vi "EXPERIMENTAL_OSCILLOSCOPE_READING.vi"() -> ()   [LabVIEW 2019]
uses:
  <instrlib>/niScope/Controls/niScope vertical coupling.ctl
  Controls/OscilloscopeBlockControl2.ctl
  Controls/DataBlockControl.ctl
  <instrlib>/niScope/Acquire/Fetch/niScope Multi Fetch Binary 16.vi
panel:
  in  "New Run?":bool=TRUE
  in  "Reset Value attempt 2":i32
  in  "Plot Data attempt 2":bool
  in  "Oscilloscope Config Cluster":T1 {"vertical coupling" items=["AC", "DC", "Ground"]}
  in  "error in":errorcluster
  in  "Oscilloscope Configuration Input Array":T1[](array[typedef]) {"vertical coupling" items=["AC", "DC", "Ground"]}
  out "Channel Graph 7":dbl[](graph)
  out "Channel Graph 6":dbl[](graph)
  out "Channel Graph 5":dbl[](graph)
  out "Channel Graph 4":dbl[](graph)
  out "Channel Graph 3":dbl[](graph)
  out "Channel Graph 2":dbl[](graph)
  out "Channel Graph 1":dbl[](graph)
  out "Channel Graph 0":dbl[](graph)
  out "Pryor's Graph":dbl[][](graph)
  in  "Plot Data":bool
  in  "Reset Value":i32=251
  in  "element":T3 {"vertical coupling" items=["AC", "DC", "Ground"]}
  in  "Oscilloscope Configuration Input Array":T4(array[cluster]) {"vertical coupling" items=["AC", "DC", "Ground"]}
  out "end record":bool
  out "error out":errorcluster
  in  "stop":bool
  out "Sample Rate IND":dbl
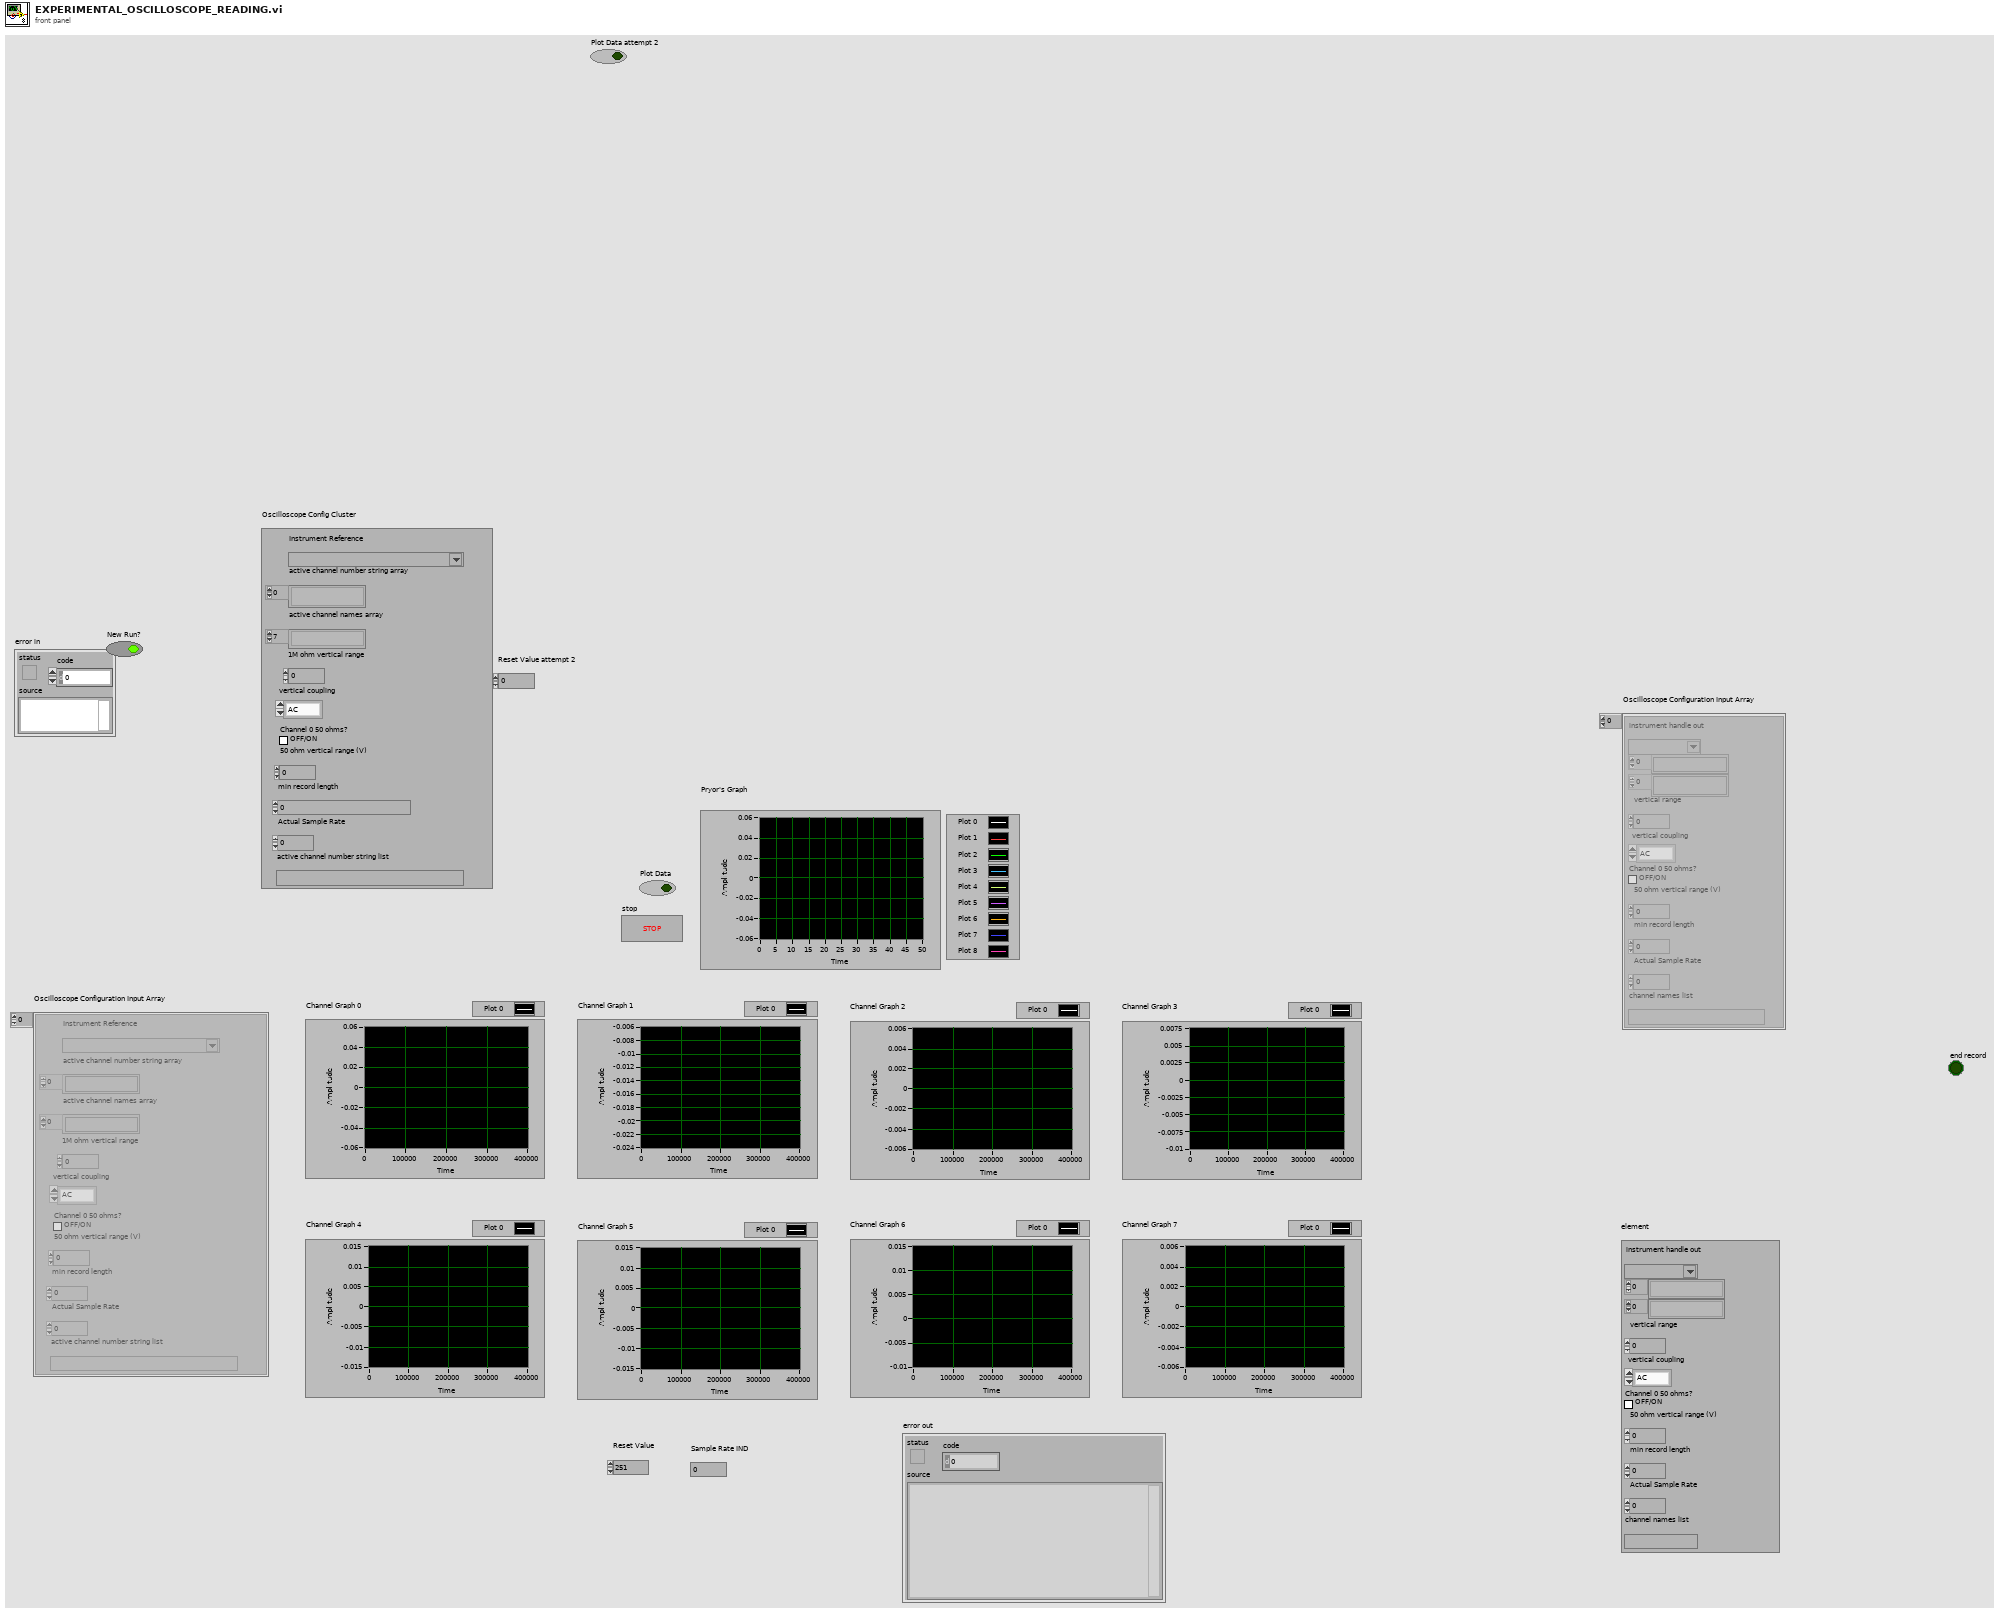
[diagram p1: front panel]
types:
  T1 = typedef "OscilloscopeBlockControl2.ctl" = cluster{"Instrument Reference":refnum<k15>, "active channel number string array":string[], "active channel names array":string[], "1M ohm vertical range":dbl, "vertical coupling":T2, "Channel 0 50 ohms?":bool, "50 ohm vertical range (V)":dbl, "min record length":i32, "Actual Sample Rate":dbl, "active channel number string list":string}
  T2 = typedef "niScope vertical coupling.ctl" = i32
  T3 = cluster{"instrument handle out":refnum<k15>, string[], string[], "vertical range":dbl, "vertical coupling":T2, "Channel 0 50 ohms?":bool, "50 ohm vertical range (V)":dbl, "min record length":i32, "Actual Sample Rate":dbl, "channel names list":string}
  T4 = cluster{"instrument handle out":refnum<k15>, string[], string[], "vertical range":dbl, "vertical coupling":T2, "Channel 0 50 ohms?":bool, "50 ohm vertical range (V)":dbl, "min record length":i32, "Actual Sample Rate":dbl, "channel names list":string}[]
  T5 = cluster{"IVI Refnum out":refnum<k15>, string, "voltage level channel 23":dbl, "Channel Name 23":string, "Current Limit":dbl, "Measure Record dt":dbl, string}[]
  T6 = typedef "DataBlockControl.ctl" = cluster{"Run Folder Parent Directory":path, "DUT":string, "Ion (ex Kr)":string, "Board Number":string, "Effective LET":string, "Test Type":enum16{"Single Event Latchup", "Single Event Transient", "Single Event Upset"}}
  T7 = enum16{"open", "replace", "create", "open or create", "replace or create", "replace or create with confirmation"}
  T8 = cluster{"Array":dbl[], "Array":dbl[], "Array":dbl[], "Array":dbl[], "Array":dbl[], "Array":dbl[], "Array":dbl[], "Array":dbl[]}
  T9 = cluster{"wfm info":cluster{"actualSamples":i32, "absoluteInitialX":dbl, "relativeInitialX":dbl, "xIncrement":dbl, "offset":dbl, "gain":dbl, "reserved1":dbl, "reserved2":dbl}[], "wfm":i16[][]}
  T10 = cluster{"created path":path, refnum<file>[], refnum<file>[]}
  T11 = enum16{"big-endian, network order", "native, host order", "little-endian"}
  T12 = cluster{"actualSamples":i32, "absoluteInitialX":dbl, "relativeInitialX":dbl, "xIncrement":dbl, "offset":dbl, "gain":dbl, "reserved1":dbl, "reserved2":dbl}[]
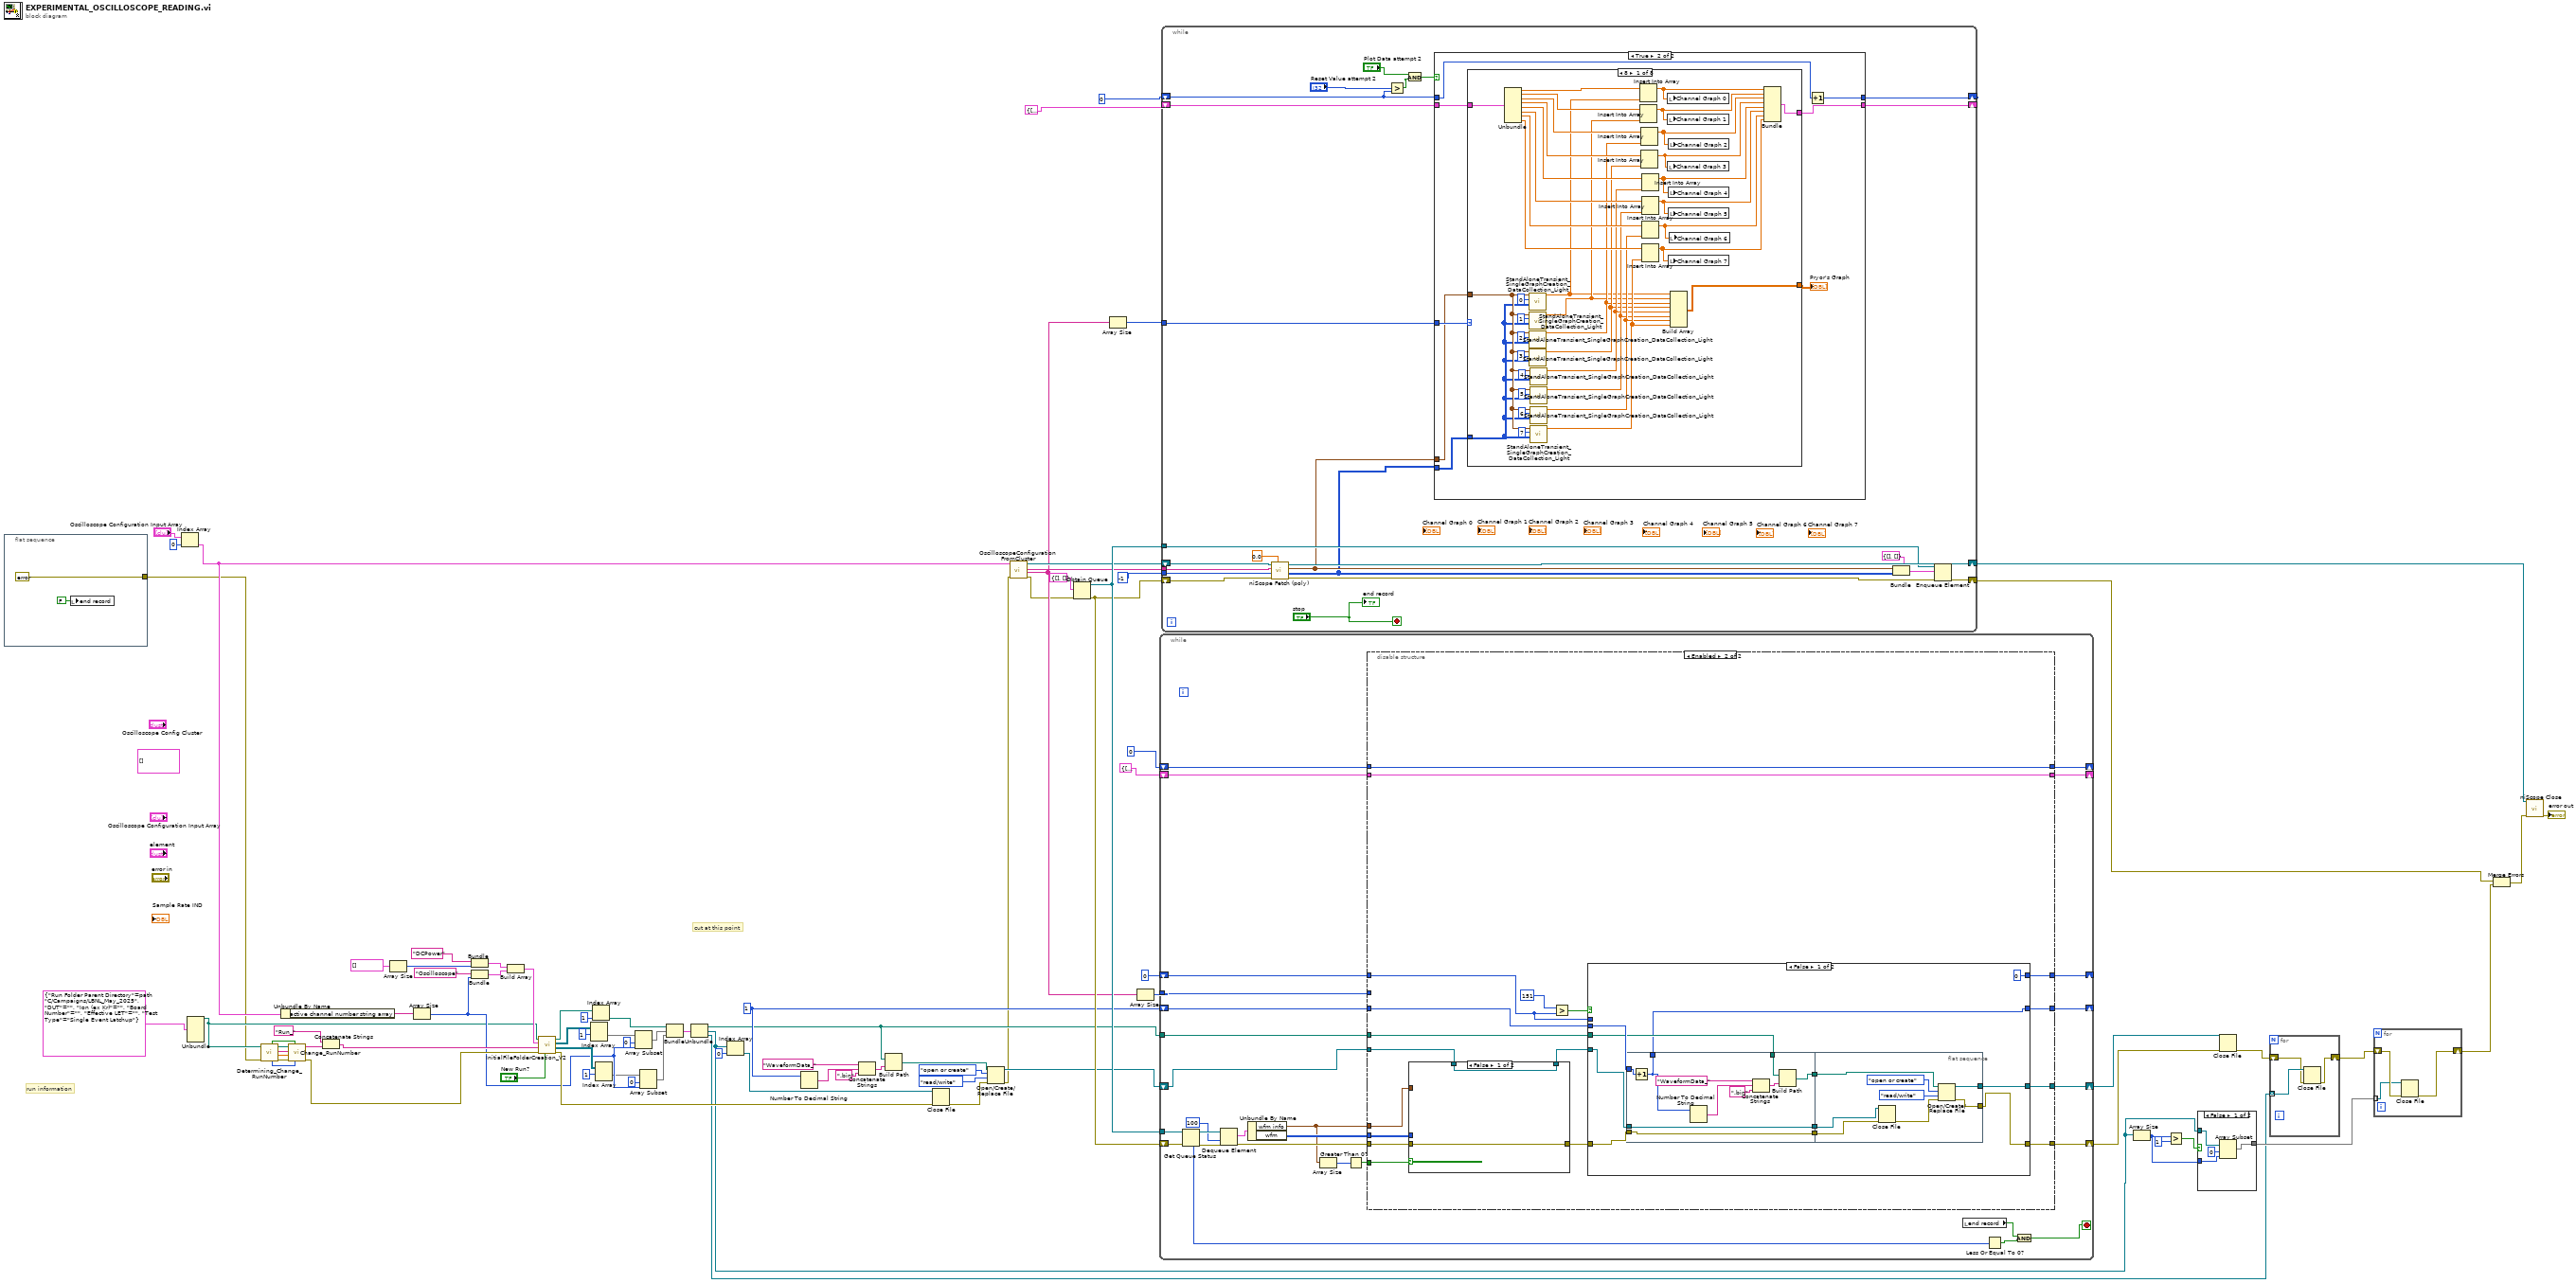
[diagram p0: block diagram]
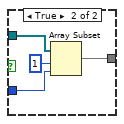
[diagram p2: hidden frame]
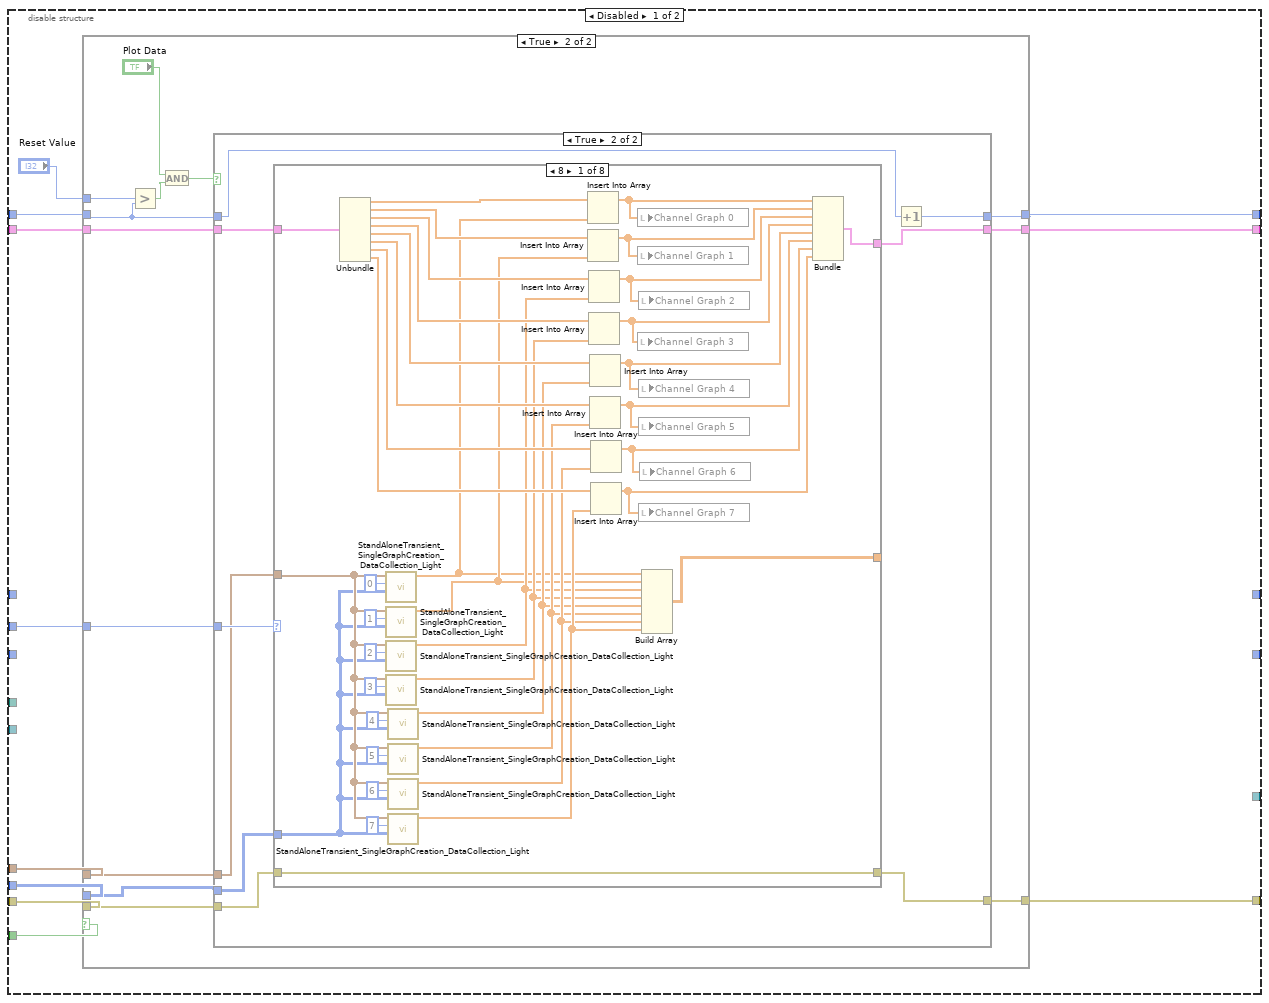
[diagram p3: hidden frame]
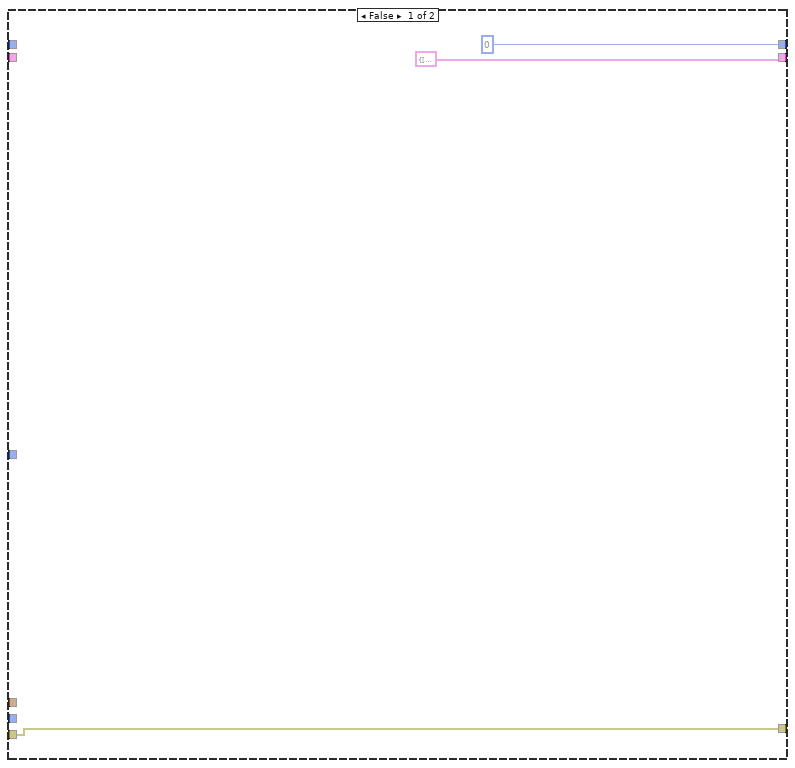
[diagram p5: hidden frame]
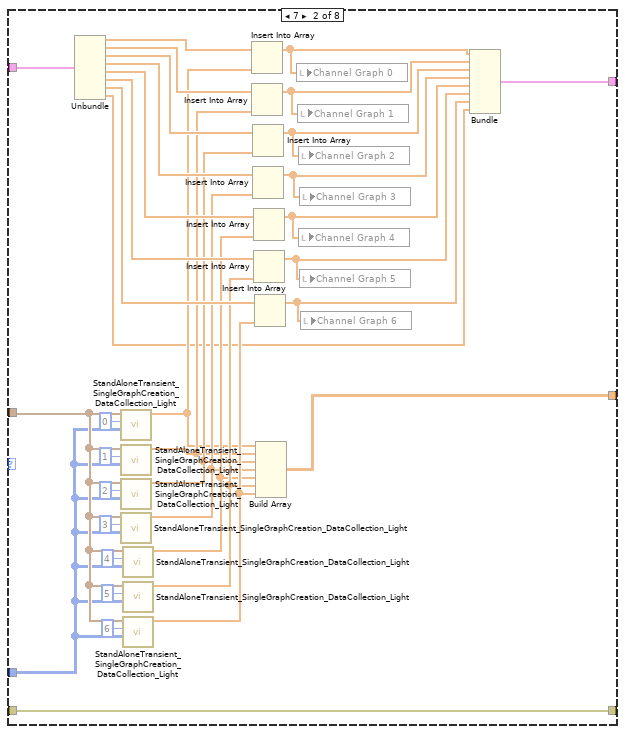
[diagram p6: hidden frame]
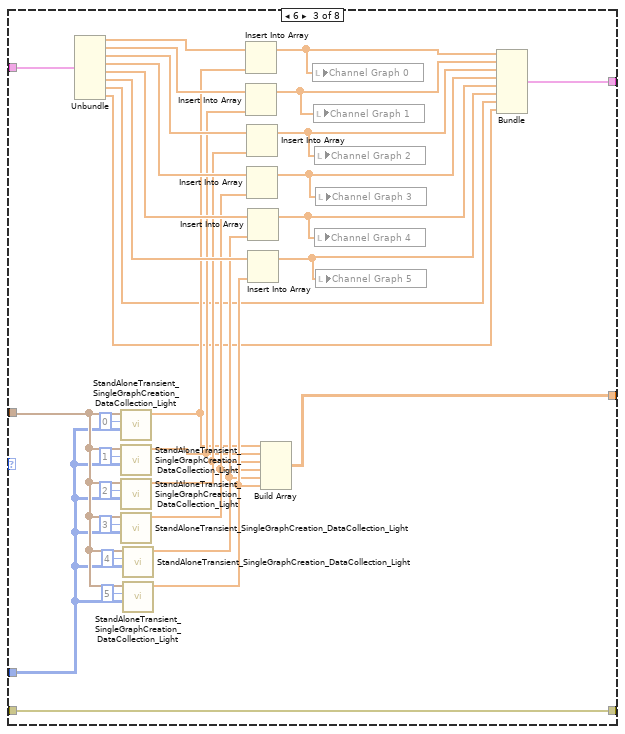
[diagram p7: hidden frame]
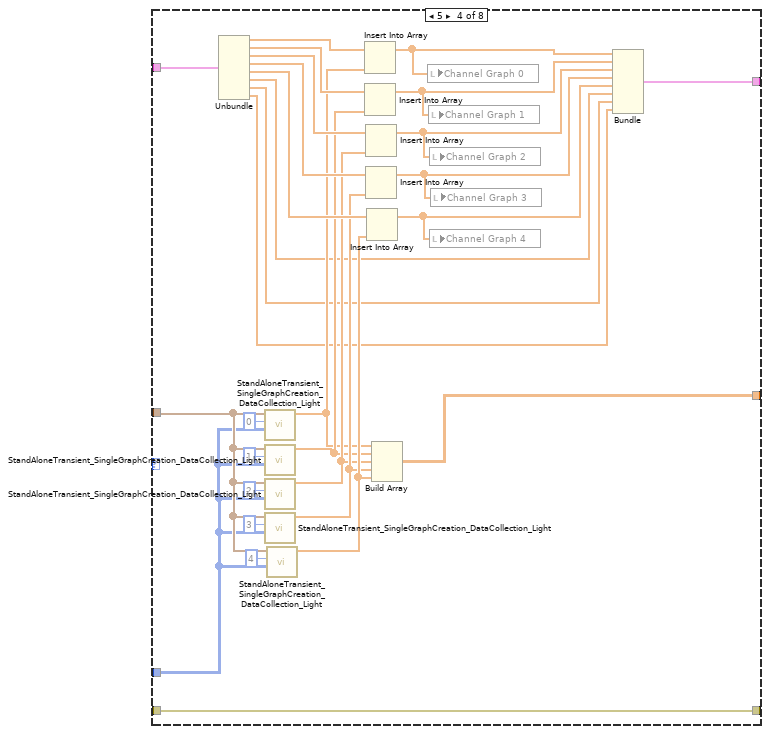
[diagram p8: hidden frame]
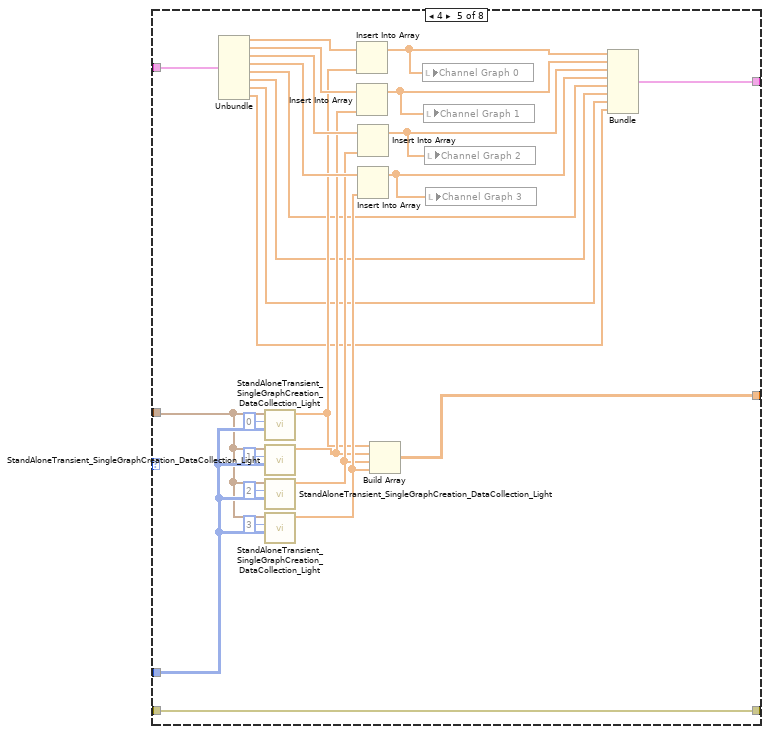
[diagram p9: hidden frame]
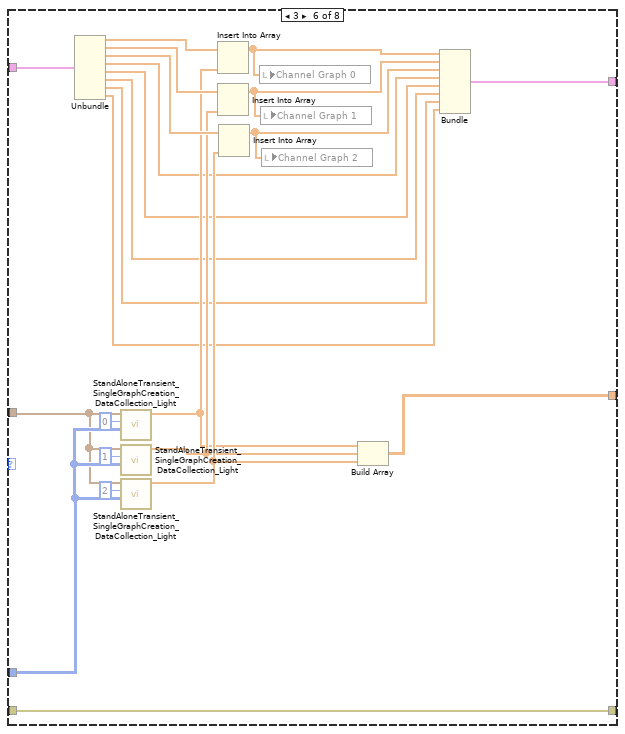
[diagram p10: hidden frame]
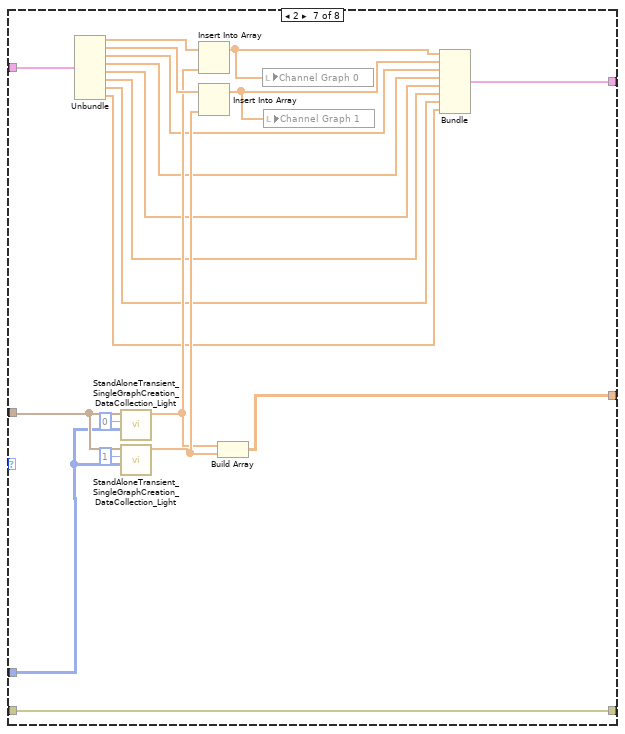
[diagram p11: hidden frame]
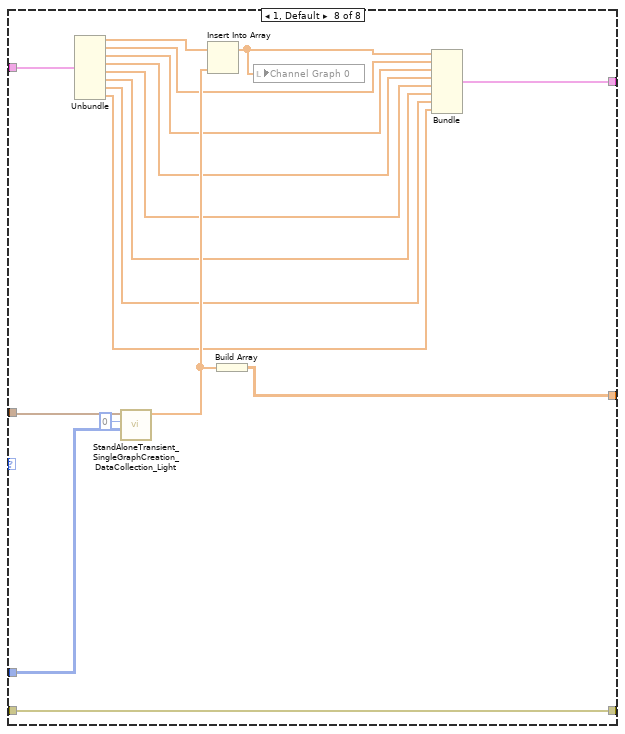
[diagram p12: hidden frame]
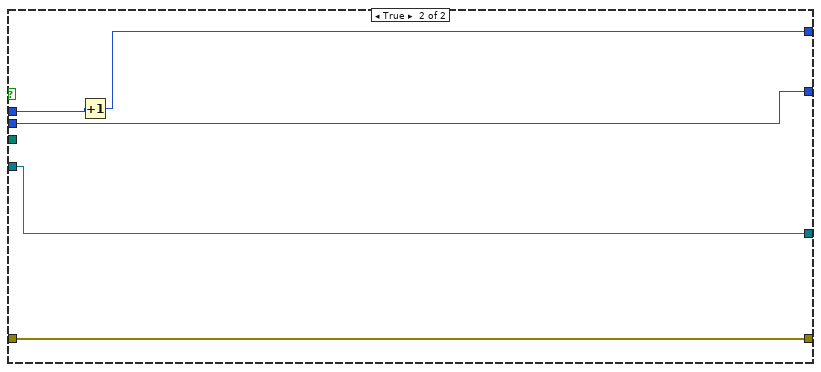
[diagram p13: hidden frame]
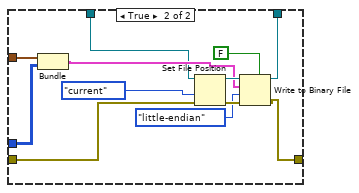
[diagram p14: hidden frame]
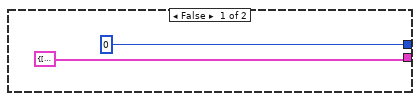
[diagram p15: hidden frame]
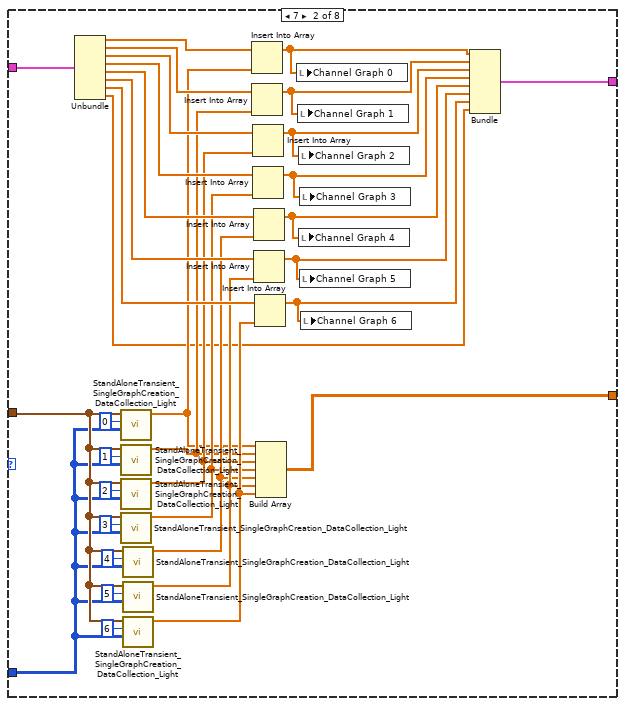
[diagram p16: hidden frame]
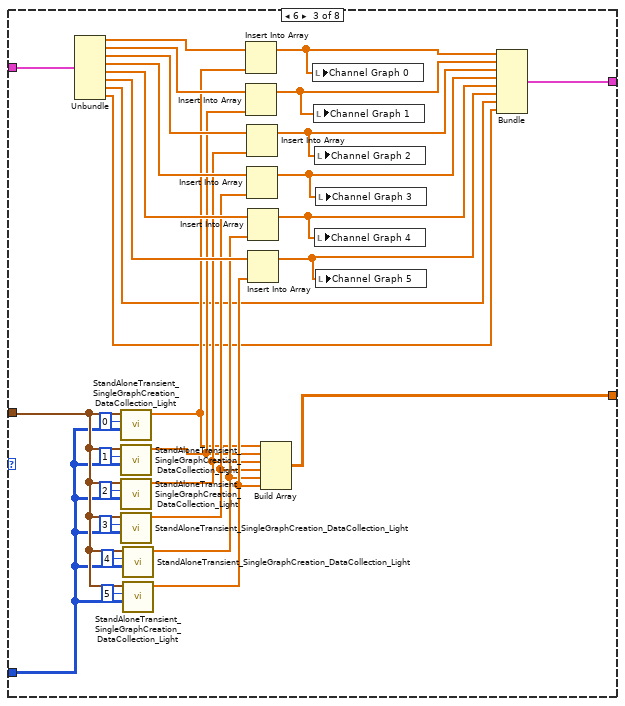
[diagram p17: hidden frame]
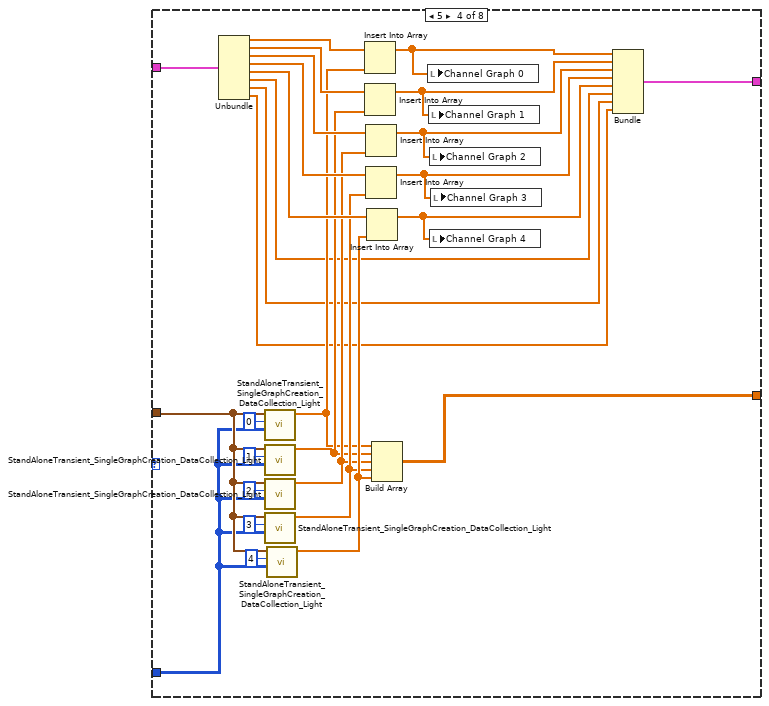
[diagram p18: hidden frame]
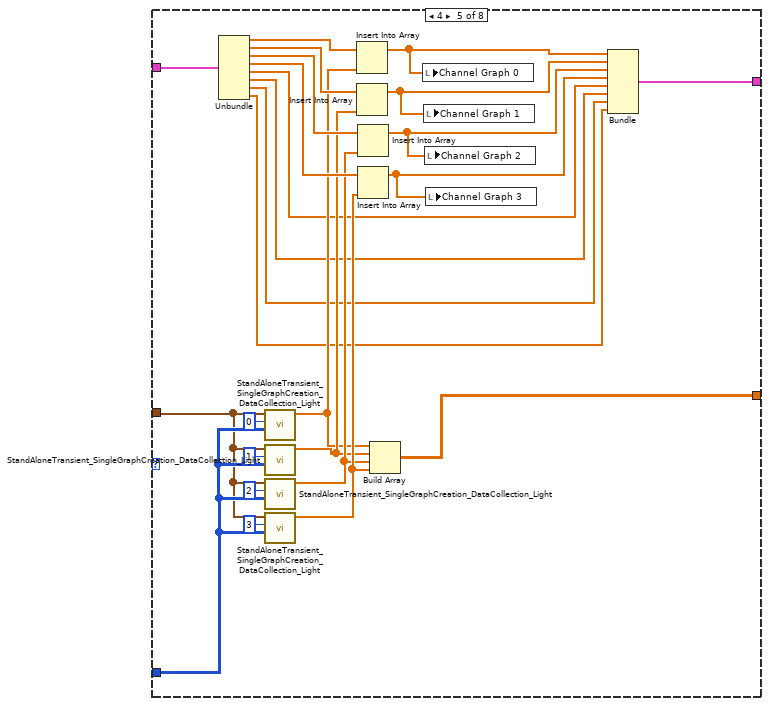
[diagram p19: hidden frame]
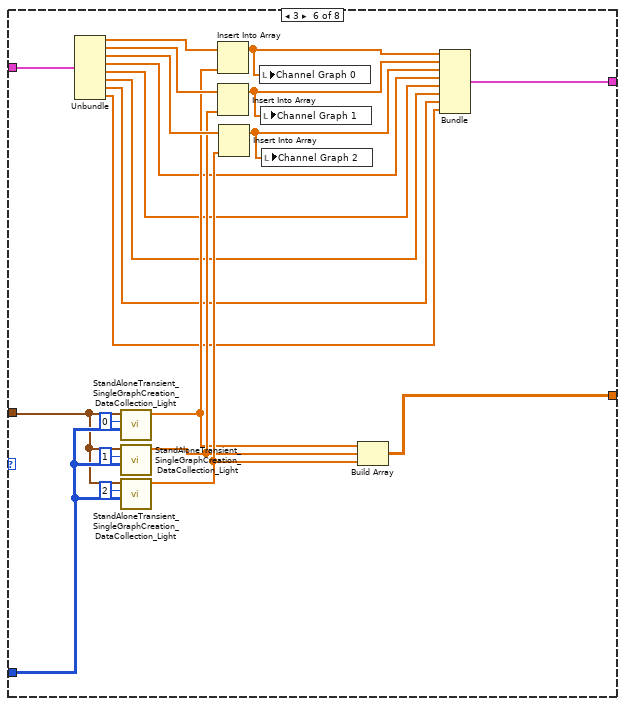
[diagram p20: hidden frame]
diagram:
  w56 = 1
  (unwired) T1[] []
  # "cut at this point"
  # "run information"
  n1 = flat-sequence {
    tunnel: [errorcluster {"status"=FALSE, "code"=0, "source"=""} ("error in")] -> w4
    frame #0 {
      n2 = local write "end record"(FALSE ("end record")) -> ()
    }
  }
  n3 = Index Array(array="Oscilloscope Configuration Input Array", index=0) -> (element=w45:T1)
  n4 = Unbundle(T6 {"Run Folder Parent Directory"=path "C:/Campaigns/LBNL_May_2025", "DUT"="", "Ion (ex Kr)"="", "Board Number"="", "Effective LET"="", "Test Type"=enum."Single Event Latchup"} ("Run Data SubPanel out")) -> ("Run Folder Parent Directory"=w18:path)  [unwired: 5 out]
  n5 = call "Determining_Change_RunNumber.vi"("error in"=w4, "Run Folder Parent Directory"=w18) -> ("error out"=w49:errorcluster, "Array"=w50:dbl[], "String"=w51:string, "path out"=w52:path, "Proposed Run Number"=w48:i32, "T button?"=w53:bool)  [unwired: 4 in]
  n6 = Unbundle By Name(w45) -> ("active channel number string array"=w39:string[])
  n7 = call "Change_RunNumber.vi"("Valid Run Number"=w48, "Changing the run number?"=w53, "error in (no error)"=w49, "Array"=w50, "String in"=w51, "path in"=w52) -> ("error out"=w35:errorcluster, "String out"=w46:string)  [unwired: 4 in]
  n8 = Concatenate Strings("Run_", w46) -> (w44:string)
  n9 = Array Size(array=T5 [] ("DCPowerInformation_byChannel")) -> (size(s)=w37:i32)
  n10 = Array Size(array=w39) -> (size(s)=w22:i32)
  n11 = Bundle("subfolder"="DCPower", w37) -> (w41:cluster{"subfolder":string, i32})  [unwired: 1 in]
  n12 = Bundle("subfolder"="Oscilloscope", w22) -> (w40:cluster{"subfolder":string, i32})  [unwired: 1 in]
  n13 = Build Array(w41, w40) -> (w36:cluster{"subfolder":string, i32}[])
  n14 = call "InitialFileFolderCreation_V2.vi"("New Run?"="New Run?", "error in (no error)"=w35, "Run Number"=w44, "Subfolders&NumChannelsRecorded"=w36, "base path"=w18) -> ("error out"=w34:errorcluster, "SupplementalDataFileReferenceObjectArrayWsubfolders"=w30:refnum<file>[][], "DataFileReferenceObjectArrayWsubfolders"=w31:refnum<file>[][], "created path array"=w32:path[])  [unwired: 3 in]
  n15 = Index Array(array=w31, index (row)=1) -> (element=w26:refnum<file>[])  [unwired: 1 in]
  n16 = Index Array(array=w32, index=1) -> (element=w29:path)
  n17 = Index Array(array=w30, index (row)=1) -> (element=w21:refnum<file>[])  [unwired: 1 in]
  n18 = Array Subset(array=w26, index=0, length=w22) -> (w28:refnum<file>[])
  n19 = Array Subset(array=w21, index=0, length=w22) -> (w27:refnum<file>[])
  n20 = Bundle("created path"=w29, w28, w27) -> (w1:T10)  [unwired: 1 in]
  n21 = Unbundle(w1) -> ("created path"=w55:path, w8:refnum<file>[], w9:refnum<file>[])
  n22 = Index Array(array=w8, index=0) -> (element=w57:refnum<file>)
  n23 = Number To Decimal String(number=w56) -> (decimal integer string=w63:string)  [unwired: 1 in]
  n24 = Concatenate Strings("WaveformData_", w63, ".bin" ("string")) -> (w62:string)
  n25 = Build Path(base path=w55, name or relative path=w62) -> (appended path=w65:path)
  n26 = Close File(refnum=w57, error in=w34) -> (error out=w58:errorcluster)  [unwired: 1 out]
  n27 = Open/Create/Replace File(file path (use dialog)=w65, error in=w58, operation (0:open)=T7."open or create", access (0:read/write)=enum16{"read/write", "read-only", "write-only"}."read/write") -> (refnum out=w7:refnum<file>, error out=w3:errorcluster)  [unwired: 2 in, 1 out]
  n28 = call "OscilloscopeConfigurationFromCluster.vi"("error in (no error)"=w3, "output cluster"=w45) -> ("error out"=w2:errorcluster, "active channel number string array"=w68:string[], "active channel number string list"=w74:string, "IVI Refnum out"=w72:refnum<k15>)  [unwired: 6 in]
  n29 = Obtain Queue(element data type=T9 {"wfm info"=[], "wfm"=[]} ("cluster"), error in (no error)=w2) -> (queue out=w81:refnum<queue>, error out=w71:errorcluster)  [unwired: 3 in, 1 out]
  n30 = Array Size(array=w68) -> (size(s)=w69:i32)
  n31 = Array Size(array=w68) -> (size(s)=w76:i32)
  n32 = while {
    shift-right: [w109] -> w11
    shift-left: w71 -> [w112]
    tunnel: w81 -> [w111]
    shift-right: [w107] -> _
    shift-left: 0 ("x") -> [w108]
    tunnel: w76 -> [w106]
    shift-right: [w105] -> _
    shift-left: T8 {"Array"=[], "Array"=[], "Array"=[], "Array"=[], "Array"=[], "Array"=[], "Array"=[], "Array"=[]} -> [w104]
    shift-right: [w93] -> _
    shift-left: w56 -> [w94]
    tunnel: w55 -> [w92]
    shift-right: [w91] -> w6
    shift-left: w7 -> [w90]
    shift-right: [w88] -> _
    shift-left: 0 ("y") -> [w89]
    stop <- w96 stop-if-true
    n33 = Get Queue Status(queue=w111, error in (no error)=w112) -> (queue out=w114:refnum<queue>, error out=w115:errorcluster, # elements in queue=w95:i32)  [unwired: 1 in, 5 out]
    n34 = Dequeue Element(queue=w114, timeout in ms (-1)=100, error in (no error)=w115) -> (element=w102:T9, error out=w110:errorcluster)  [unwired: 2 out]
    n35 = Unbundle By Name(w102) -> ("wfm info"=w101:T12, "wfm"=w103:i16[][])
    n36 = Array Size(array=w101) -> (size(s)=w100:i32)
    n37 = Greater Than 0?(x=w100) -> (x > 0?=w99:bool)
    n38 = disable-structure shown="Enabled" {
      disable-tunnel: w110 -> [w126 w390]
      disable-tunnel: [w125 w386] -> w109
      disable-tunnel: w108 -> [w123 w391]
      disable-tunnel: [w122 w391] -> w107
      disable-tunnel: w106 -> [w121 _]
      disable-tunnel: [w120 w392] -> w105
      disable-tunnel: w104 -> [w119 w392]
      disable-tunnel: w103 -> [w118 w388]
      disable-tunnel: w101 -> [w117 w389]
      disable-tunnel: w99 -> [w116 w387]
      disable-tunnel: w94 -> [_ w382]
      disable-tunnel: [_ w384] -> w93
      disable-tunnel: w90 -> [_ w379]
      disable-tunnel: w92 -> [_ w380]
      disable-tunnel: [_ w377] -> w91
      disable-tunnel: w89 -> [_ w376]
      disable-tunnel: [_ w375] -> w88
      frame Disabled {
        n39 = case shown="True" w116 {
          tunnel: w126 -> [w129 w142]
          tunnel: [w129 w141] -> w125
          tunnel: "Reset Value" -> [_ w140]
          tunnel: w123 -> [w128 w139]
          tunnel: [w128 w138] -> w122
          tunnel: w121 -> [_ w136]
          tunnel: [w127 w135] -> w120
          tunnel: w119 -> [w127 w134]
          tunnel: w117 -> [_ w131]
          tunnel: w118 -> [_ w130]
          frame False {
          }
          frame True {
            n40 = Greater?(x=w140, y=w139) -> (0:w132:bool)
            n41 = And(x="Plot Data", y=w132) -> (x .and. y?=w133:bool)
            n42 = case shown="True" w133 {
              tunnel: w136 -> [_ w154]
              tunnel: w131 -> [_ w153]
              tunnel: w130 -> [_ w152]
              tunnel: w142 -> [w143 w151]
              tunnel: [T8 {"Array"=[], "Array"=[], "Array"=[], "Array"=[], "Array"=[], "Array"=[], "Array"=[], "Array"=[]} w150] -> w135
              tunnel: w134 -> [_ w149]
              tunnel: [w143 w148] -> w141
              tunnel: [0 ("x") w147] -> w138
              tunnel: w139 -> [_ w146]
              frame False {
              }
              frame True {
                n43 = case shown="8" w154 {
                  tunnel: w153 -> [w192 w227 w259 w288 w289 w315 w357 w374]
                  tunnel: w152 -> [w191 w226 w258 w287 w314 w337 w356 w373]
                  tunnel: [w182 w218 w251 w281 w309 w333 w353 w371] -> _
                  tunnel: [w181 w217 w250 w280 w308 w332 w352 w370] -> w148
                  tunnel: w151 -> [w181 w217 w250 w280 w308 w332 w352 w370]
                  tunnel: [w180 w216 w249 w279 w307 w331 w351 w369] -> w150
                  tunnel: w149 -> [w179 w215 w248 w278 w306 w330 w350 w368]
                  frame 8 {
                    n44 = Unbundle(w179) -> ("Array"=w178:dbl[], "Array"=w177:dbl[], "Array"=w176:dbl[], "Array"=w175:dbl[], "Array"=w174:dbl[], "Array"=w173:dbl[], "Array"=w172:dbl[], "Array"=w171:dbl[])
                    n45 = call "StandAloneTransient_SingleGraphCreation_DataCollection_Light.vi"("wfm"=w191, "index"=0, "wfm info"=w192) -> ("Array"=w163:dbl[])  [unwired: 8 in]
                    n46 = call "StandAloneTransient_SingleGraphCreation_DataCollection_Light.vi"("wfm"=w191, "index"=1, "wfm info"=w192) -> ("Array"=w164:dbl[])  [unwired: 8 in]
                    n47 = call "StandAloneTransient_SingleGraphCreation_DataCollection_Light.vi"("wfm"=w191, "index"=2, "wfm info"=w192) -> ("Array"=w165:dbl[])  [unwired: 8 in]
                    n48 = call "StandAloneTransient_SingleGraphCreation_DataCollection_Light.vi"("wfm"=w191, "index"=3, "wfm info"=w192) -> ("Array"=w166:dbl[])  [unwired: 8 in]
                    n49 = call "StandAloneTransient_SingleGraphCreation_DataCollection_Light.vi"("wfm"=w191, "index"=4, "wfm info"=w192) -> ("Array"=w167:dbl[])  [unwired: 8 in]
                    n50 = call "StandAloneTransient_SingleGraphCreation_DataCollection_Light.vi"("wfm"=w191, "index"=5, "wfm info"=w192) -> ("Array"=w168:dbl[])  [unwired: 8 in]
                    n51 = call "StandAloneTransient_SingleGraphCreation_DataCollection_Light.vi"("wfm"=w191, "index"=6, "wfm info"=w192) -> ("Array"=w169:dbl[])  [unwired: 8 in]
                    n52 = call "StandAloneTransient_SingleGraphCreation_DataCollection_Light.vi"("wfm"=w191, "index"=7, "wfm info"=w192) -> ("Array"=w170:dbl[])  [unwired: 8 in]
                    n53 = Insert Into Array(array=w178, new element=w163) -> (w162:dbl[])  [unwired: 1 in]
                    n54 = Insert Into Array(array=w177, new element=w164) -> (w161:dbl[])  [unwired: 1 in]
                    n55 = Insert Into Array(array=w176, new element=w165) -> (w160:dbl[])  [unwired: 1 in]
                    n56 = Insert Into Array(array=w175, new element=w166) -> (w159:dbl[])  [unwired: 1 in]
                    n57 = Insert Into Array(array=w174, new element=w167) -> (w158:dbl[])  [unwired: 1 in]
                    n58 = Insert Into Array(array=w173, new element=w168) -> (w157:dbl[])  [unwired: 1 in]
                    n59 = Insert Into Array(array=w172, new element=w169) -> (w156:dbl[])  [unwired: 1 in]
                    n60 = Insert Into Array(array=w171, new element=w170) -> (w155:dbl[])  [unwired: 1 in]
                    n61 = local write "Channel Graph 0"(w162) -> ()
                    n62 = local write "Channel Graph 1"(w161) -> ()
                    n63 = local write "Channel Graph 3"(w159) -> ()
                    n64 = local write "Channel Graph 2"(w160) -> ()
                    n65 = local write "Channel Graph 4"(w158) -> ()
                    n66 = local write "Channel Graph 5"(w157) -> ()
                    n67 = local write "Channel Graph 7"(w155) -> ()
                    n68 = local write "Channel Graph 6"(w156) -> ()
                    n69 = Build Array(w163, w164, w165, w166, w167, w168, w169, w170) -> (w182:dbl[][])
                    n70 = Bundle("Array"=w162, "Array"=w161, "Array"=w160, "Array"=w159, "Array"=w158, "Array"=w157, "Array"=w156, "Array"=w155) -> (w180:T8)  [unwired: 1 in]
                  }
                  frame 7 {
                    n71 = Unbundle(w215) -> ("Array"=w214:dbl[], "Array"=w213:dbl[], "Array"=w212:dbl[], "Array"=w211:dbl[], "Array"=w210:dbl[], "Array"=w209:dbl[], "Array"=w208:dbl[], "Array"=w193:dbl[])
                    n72 = call "StandAloneTransient_SingleGraphCreation_DataCollection_Light.vi"("wfm"=w226, "index"=0, "wfm info"=w227) -> ("Array"=w201:dbl[])  [unwired: 8 in]
                    n73 = call "StandAloneTransient_SingleGraphCreation_DataCollection_Light.vi"("wfm"=w226, "index"=1, "wfm info"=w227) -> ("Array"=w202:dbl[])  [unwired: 8 in]
                    n74 = call "StandAloneTransient_SingleGraphCreation_DataCollection_Light.vi"("wfm"=w226, "index"=2, "wfm info"=w227) -> ("Array"=w203:dbl[])  [unwired: 8 in]
                    n75 = call "StandAloneTransient_SingleGraphCreation_DataCollection_Light.vi"("wfm"=w226, "index"=3, "wfm info"=w227) -> ("Array"=w204:dbl[])  [unwired: 8 in]
                    n76 = call "StandAloneTransient_SingleGraphCreation_DataCollection_Light.vi"("wfm"=w226, "index"=4, "wfm info"=w227) -> ("Array"=w205:dbl[])  [unwired: 8 in]
                    n77 = call "StandAloneTransient_SingleGraphCreation_DataCollection_Light.vi"("wfm"=w226, "index"=5, "wfm info"=w227) -> ("Array"=w206:dbl[])  [unwired: 8 in]
                    n78 = call "StandAloneTransient_SingleGraphCreation_DataCollection_Light.vi"("wfm"=w226, "index"=6, "wfm info"=w227) -> ("Array"=w207:dbl[])  [unwired: 8 in]
                    n79 = Insert Into Array(array=w214, new element=w201) -> (w200:dbl[])  [unwired: 1 in]
                    n80 = Insert Into Array(array=w213, new element=w202) -> (w199:dbl[])  [unwired: 1 in]
                    n81 = Insert Into Array(array=w212, new element=w203) -> (w198:dbl[])  [unwired: 1 in]
                    n82 = Insert Into Array(array=w211, new element=w204) -> (w197:dbl[])  [unwired: 1 in]
                    n83 = Insert Into Array(array=w210, new element=w205) -> (w196:dbl[])  [unwired: 1 in]
                    n84 = Insert Into Array(array=w209, new element=w206) -> (w195:dbl[])  [unwired: 1 in]
                    n85 = Insert Into Array(array=w208, new element=w207) -> (w194:dbl[])  [unwired: 1 in]
                    n86 = Build Array(w201, w202, w203, w204, w205, w206, w207) -> (w218:dbl[][])
                    n87 = local write "Channel Graph 0"(w200) -> ()
                    n88 = local write "Channel Graph 1"(w199) -> ()
                    n89 = local write "Channel Graph 2"(w198) -> ()
                    n90 = local write "Channel Graph 4"(w196) -> ()
                    n91 = local write "Channel Graph 3"(w197) -> ()
                    n92 = local write "Channel Graph 5"(w195) -> ()
                    n93 = local write "Channel Graph 6"(w194) -> ()
                    n94 = Bundle("Array"=w200, "Array"=w199, "Array"=w198, "Array"=w197, "Array"=w196, "Array"=w195, "Array"=w194, "Array"=w193) -> (w216:T8)  [unwired: 1 in]
                  }
                  frame 6 {
                    n95 = Unbundle(w248) -> ("Array"=w247:dbl[], "Array"=w246:dbl[], "Array"=w245:dbl[], "Array"=w244:dbl[], "Array"=w243:dbl[], "Array"=w242:dbl[], "Array"=w229:dbl[], "Array"=w228:dbl[])
                    n96 = call "StandAloneTransient_SingleGraphCreation_DataCollection_Light.vi"("wfm"=w258, "index"=0, "wfm info"=w259) -> ("Array"=w236:dbl[])  [unwired: 8 in]
                    n97 = call "StandAloneTransient_SingleGraphCreation_DataCollection_Light.vi"("wfm"=w258, "index"=1, "wfm info"=w259) -> ("Array"=w237:dbl[])  [unwired: 8 in]
                    n98 = call "StandAloneTransient_SingleGraphCreation_DataCollection_Light.vi"("wfm"=w258, "index"=2, "wfm info"=w259) -> ("Array"=w238:dbl[])  [unwired: 8 in]
                    n99 = call "StandAloneTransient_SingleGraphCreation_DataCollection_Light.vi"("wfm"=w258, "index"=3, "wfm info"=w259) -> ("Array"=w239:dbl[])  [unwired: 8 in]
                    n100 = call "StandAloneTransient_SingleGraphCreation_DataCollection_Light.vi"("wfm"=w258, "index"=4, "wfm info"=w259) -> ("Array"=w240:dbl[])  [unwired: 8 in]
                    n101 = call "StandAloneTransient_SingleGraphCreation_DataCollection_Light.vi"("wfm"=w258, "index"=5, "wfm info"=w259) -> ("Array"=w241:dbl[])  [unwired: 8 in]
                    n102 = Insert Into Array(array=w247, new element=w236) -> (w235:dbl[])  [unwired: 1 in]
                    n103 = Insert Into Array(array=w246, new element=w237) -> (w234:dbl[])  [unwired: 1 in]
                    n104 = Insert Into Array(array=w245, new element=w238) -> (w233:dbl[])  [unwired: 1 in]
                    n105 = Insert Into Array(array=w244, new element=w239) -> (w232:dbl[])  [unwired: 1 in]
                    n106 = Insert Into Array(array=w243, new element=w240) -> (w231:dbl[])  [unwired: 1 in]
                    n107 = Insert Into Array(array=w242, new element=w241) -> (w230:dbl[])  [unwired: 1 in]
                    n108 = Build Array(w236, w237, w238, w239, w240, w241) -> (w251:dbl[][])
                    n109 = local write "Channel Graph 0"(w235) -> ()
                    n110 = local write "Channel Graph 1"(w234) -> ()
                    n111 = local write "Channel Graph 2"(w233) -> ()
                    n112 = local write "Channel Graph 4"(w231) -> ()
                    n113 = local write "Channel Graph 3"(w232) -> ()
                    n114 = local write "Channel Graph 5"(w230) -> ()
                    n115 = Bundle("Array"=w235, "Array"=w234, "Array"=w233, "Array"=w232, "Array"=w231, "Array"=w230, "Array"=w229, "Array"=w228) -> (w249:T8)  [unwired: 1 in]
                  }
                  frame 5 {
                    n116 = Unbundle(w278) -> ("Array"=w277:dbl[], "Array"=w276:dbl[], "Array"=w275:dbl[], "Array"=w274:dbl[], "Array"=w273:dbl[], "Array"=w262:dbl[], "Array"=w261:dbl[], "Array"=w260:dbl[])
                    n117 = call "StandAloneTransient_SingleGraphCreation_DataCollection_Light.vi"("wfm"=w287, "index"=0, "wfm info"=w288) -> ("Array"=w268:dbl[])  [unwired: 8 in]
                    n118 = call "StandAloneTransient_SingleGraphCreation_DataCollection_Light.vi"("wfm"=w287, "index"=1, "wfm info"=w288) -> ("Array"=w269:dbl[])  [unwired: 8 in]
                    n119 = call "StandAloneTransient_SingleGraphCreation_DataCollection_Light.vi"("wfm"=w287, "index"=2, "wfm info"=w288) -> ("Array"=w270:dbl[])  [unwired: 8 in]
                    n120 = call "StandAloneTransient_SingleGraphCreation_DataCollection_Light.vi"("wfm"=w287, "index"=3, "wfm info"=w288) -> ("Array"=w271:dbl[])  [unwired: 8 in]
                    n121 = call "StandAloneTransient_SingleGraphCreation_DataCollection_Light.vi"("wfm"=w287, "index"=4, "wfm info"=w288) -> ("Array"=w272:dbl[])  [unwired: 8 in]
                    n122 = Insert Into Array(array=w277, new element=w268) -> (w267:dbl[])  [unwired: 1 in]
                    n123 = Insert Into Array(array=w276, new element=w269) -> (w266:dbl[])  [unwired: 1 in]
                    n124 = Insert Into Array(array=w275, new element=w270) -> (w265:dbl[])  [unwired: 1 in]
                    n125 = Insert Into Array(array=w274, new element=w271) -> (w264:dbl[])  [unwired: 1 in]
                    n126 = Insert Into Array(array=w273, new element=w272) -> (w263:dbl[])  [unwired: 1 in]
                    n127 = Build Array(w268, w269, w270, w271, w272) -> (w281:dbl[][])
                    n128 = local write "Channel Graph 0"(w267) -> ()
                    n129 = local write "Channel Graph 1"(w266) -> ()
                    n130 = local write "Channel Graph 2"(w265) -> ()
                    n131 = local write "Channel Graph 4"(w263) -> ()
                    n132 = local write "Channel Graph 3"(w264) -> ()
                    n133 = Bundle("Array"=w267, "Array"=w266, "Array"=w265, "Array"=w264, "Array"=w263, "Array"=w262, "Array"=w261, "Array"=w260) -> (w279:T8)  [unwired: 1 in]
                  }
                  frame 4 {
                    n134 = Unbundle(w306) -> ("Array"=w305:dbl[], "Array"=w304:dbl[], "Array"=w303:dbl[], "Array"=w302:dbl[], "Array"=w293:dbl[], "Array"=w292:dbl[], "Array"=w291:dbl[], "Array"=w290:dbl[])
                    n135 = call "StandAloneTransient_SingleGraphCreation_DataCollection_Light.vi"("wfm"=w314, "index"=0, "wfm info"=w289) -> ("Array"=w298:dbl[])  [unwired: 8 in]
                    n136 = call "StandAloneTransient_SingleGraphCreation_DataCollection_Light.vi"("wfm"=w314, "index"=1, "wfm info"=w289) -> ("Array"=w299:dbl[])  [unwired: 8 in]
                    n137 = call "StandAloneTransient_SingleGraphCreation_DataCollection_Light.vi"("wfm"=w314, "index"=2, "wfm info"=w289) -> ("Array"=w300:dbl[])  [unwired: 8 in]
                    n138 = call "StandAloneTransient_SingleGraphCreation_DataCollection_Light.vi"("wfm"=w314, "index"=3, "wfm info"=w289) -> ("Array"=w301:dbl[])  [unwired: 8 in]
                    n139 = Insert Into Array(array=w305, new element=w298) -> (w297:dbl[])  [unwired: 1 in]
                    n140 = Insert Into Array(array=w304, new element=w299) -> (w296:dbl[])  [unwired: 1 in]
                    n141 = Insert Into Array(array=w303, new element=w300) -> (w295:dbl[])  [unwired: 1 in]
                    n142 = Insert Into Array(array=w302, new element=w301) -> (w294:dbl[])  [unwired: 1 in]
                    n143 = Build Array(w298, w299, w300, w301) -> (w309:dbl[][])
                    n144 = local write "Channel Graph 0"(w297) -> ()
                    n145 = local write "Channel Graph 1"(w296) -> ()
                    n146 = local write "Channel Graph 2"(w295) -> ()
                    n147 = local write "Channel Graph 3"(w294) -> ()
                    n148 = Bundle("Array"=w297, "Array"=w296, "Array"=w295, "Array"=w294, "Array"=w293, "Array"=w292, "Array"=w291, "Array"=w290) -> (w307:T8)  [unwired: 1 in]
                  }
                  frame 3 {
                    n149 = Unbundle(w330) -> ("Array"=w329:dbl[], "Array"=w328:dbl[], "Array"=w327:dbl[], "Array"=w320:dbl[], "Array"=w319:dbl[], "Array"=w318:dbl[], "Array"=w317:dbl[], "Array"=w316:dbl[])
                    n150 = call "StandAloneTransient_SingleGraphCreation_DataCollection_Light.vi"("wfm"=w337, "index"=0, "wfm info"=w315) -> ("Array"=w324:dbl[])  [unwired: 8 in]
                    n151 = call "StandAloneTransient_SingleGraphCreation_DataCollection_Light.vi"("wfm"=w337, "index"=1, "wfm info"=w315) -> ("Array"=w325:dbl[])  [unwired: 8 in]
                    n152 = call "StandAloneTransient_SingleGraphCreation_DataCollection_Light.vi"("wfm"=w337, "index"=2, "wfm info"=w315) -> ("Array"=w326:dbl[])  [unwired: 8 in]
                    n153 = Insert Into Array(array=w329, new element=w324) -> (w323:dbl[])  [unwired: 1 in]
                    n154 = Insert Into Array(array=w328, new element=w325) -> (w322:dbl[])  [unwired: 1 in]
                    n155 = Insert Into Array(array=w327, new element=w326) -> (w321:dbl[])  [unwired: 1 in]
                    n156 = local write "Channel Graph 0"(w323) -> ()
                    n157 = local write "Channel Graph 1"(w322) -> ()
                    n158 = local write "Channel Graph 2"(w321) -> ()
                    n159 = Build Array(w324, w325, w326) -> (w333:dbl[][])
                    n160 = Bundle("Array"=w323, "Array"=w322, "Array"=w321, "Array"=w320, "Array"=w319, "Array"=w318, "Array"=w317, "Array"=w316) -> (w331:T8)  [unwired: 1 in]
                  }
                  frame 2 {
                    n161 = Unbundle(w350) -> ("Array"=w349:dbl[], "Array"=w348:dbl[], "Array"=w343:dbl[], "Array"=w342:dbl[], "Array"=w341:dbl[], "Array"=w340:dbl[], "Array"=w339:dbl[], "Array"=w338:dbl[])
                    n162 = call "StandAloneTransient_SingleGraphCreation_DataCollection_Light.vi"("wfm"=w356, "index"=0, "wfm info"=w357) -> ("Array"=w346:dbl[])  [unwired: 8 in]
                    n163 = call "StandAloneTransient_SingleGraphCreation_DataCollection_Light.vi"("wfm"=w356, "index"=1, "wfm info"=w357) -> ("Array"=w347:dbl[])  [unwired: 8 in]
                    n164 = Insert Into Array(array=w349, new element=w346) -> (w345:dbl[])  [unwired: 1 in]
                    n165 = Insert Into Array(array=w348, new element=w347) -> (w344:dbl[])  [unwired: 1 in]
                    n166 = Build Array(w346, w347) -> (w353:dbl[][])
                    n167 = local write "Channel Graph 0"(w345) -> ()
                    n168 = local write "Channel Graph 1"(w344) -> ()
                    n169 = Bundle("Array"=w345, "Array"=w344, "Array"=w343, "Array"=w342, "Array"=w341, "Array"=w340, "Array"=w339, "Array"=w338) -> (w351:T8)  [unwired: 1 in]
                  }
                  frame 1, Default {
                    n170 = Unbundle(w368) -> ("Array"=w367:dbl[], "Array"=w364:dbl[], "Array"=w363:dbl[], "Array"=w362:dbl[], "Array"=w361:dbl[], "Array"=w360:dbl[], "Array"=w359:dbl[], "Array"=w358:dbl[])
                    n171 = call "StandAloneTransient_SingleGraphCreation_DataCollection_Light.vi"("wfm"=w373, "index"=0, "wfm info"=w374) -> ("Array"=w366:dbl[])  [unwired: 8 in]
                    n172 = Insert Into Array(array=w367, new element=w366) -> (w365:dbl[])  [unwired: 1 in]
                    n173 = Build Array(w366) -> (w371:dbl[][])
                    n174 = local write "Channel Graph 0"(w365) -> ()
                    n175 = Bundle("Array"=w365, "Array"=w364, "Array"=w363, "Array"=w362, "Array"=w361, "Array"=w360, "Array"=w359, "Array"=w358) -> (w369:T8)  [unwired: 1 in]
                  }
                }
                n176 = Increment(x=w146) -> (x+1=w147:i32)
              }
            }
          }
        }
      }
      frame Enabled {
        n177 = case shown="False" w387 {
          tunnel: w390 -> [w428 w435]
          tunnel: [w428 w434] -> w385
          tunnel: w389 -> [_ w432]
          tunnel: w388 -> [_ w431]
          tunnel: w379 -> [w427 w430]
          tunnel: [w427 w429] -> w378
          frame False {
          }
          frame True {
            n178 = Bundle("wfm info"=w432, "wfm"=w431) -> (w433:T9)  [unwired: 1 in]
            n179 = Set File Position(refnum=w430, from (0:start)=enum16{"start", "end", "current"}."current", error in=w435) -> (refnum out=w439:refnum<file>, error out=w440:errorcluster)  [unwired: 1 in]
            n180 = Write to Binary File(file (use dialog)=w439, data=w433, error in=w440, 5:FALSE ("prepend array or string size? (T)"), 9:T11."little-endian" ("byte order (0:big-endian, network order)")) -> (refnum out=w429:refnum<file>, error out=w434:errorcluster)  [unwired: 1 in, 1 out]
          }
        }
        n181 = Greater?(x=151, y=w376) -> (0:w383:bool)
        n182 = case shown="False" w383 {
          tunnel: [w399 w426] -> w386
          tunnel: w385 -> [w400 w426]
          tunnel: w382 -> [w398 w424]
          tunnel: [w394 w424] -> w384
          tunnel: w378 -> [w397 w425]
          tunnel: w380 -> [w396 _]
          tunnel: [w395 w425] -> w377
          tunnel: w376 -> [_ w423]
          tunnel: [0 w422] -> w375
          frame False {
            n183 = flat-sequence {
              tunnel: w400 -> [w410]
              tunnel: [w410] -> w403
              tunnel: [w409] -> w402
              tunnel: [w408] -> w401
              tunnel: w397 -> [w408]
              tunnel: w396 -> [w406]
              tunnel: w398 -> [w405]
              tunnel: [w404] -> w394
              tunnel: w403 -> [w415]
              tunnel: w402 -> [w418]
              tunnel: [w417] -> w395
              tunnel: [w416] -> w399
              tunnel: w401 -> [w414]
              frame #0 {
                n184 = Increment(x=w405) -> (x+1=w404:i32)
                n185 = Number To Decimal String(number=w404) -> (decimal integer string=w412:string)  [unwired: 1 in]
                n186 = Concatenate Strings("WaveformData_", w412, ".bin" ("string")) -> (w411:string)
                n187 = Build Path(base path=w406, name or relative path=w411) -> (appended path=w409:path)
              }
              frame #1 {
                n188 = Close File(refnum=w414, error in=w415) -> (error out=w419:errorcluster)  [unwired: 1 out]
                n189 = Open/Create/Replace File(file path (use dialog)=w418, error in=w419, operation (0:open)=T7."open or create", access (0:read/write)=enum16{"read/write", "read-only", "write-only"}."read/write") -> (refnum out=w417:refnum<file>, error out=w416:errorcluster)  [unwired: 2 in, 1 out]
              }
            }
          }
          frame True {
            n190 = Increment(x=w423) -> (x+1=w422:i32)
          }
        }
      }
    }
    n191 = local read "end record"() -> (w97:bool)
    n192 = Less Or Equal To 0?(x=w95) -> (x <= 0?=w98:bool)
    n193 = And(x=w97, y=w98) -> (x .and. y?=w96:bool)
  }
  n194 = while {
    shift-right: [w461] -> w84
    shift-left: w72 -> [w463]
    shift-right: [w452] -> w79
    shift-left: w71 -> [w462]
    tunnel: w74 -> [w459]
    tunnel: -1 ("numSamples") -> [w458]
    tunnel: w81 -> [w455]
    tunnel: w69 -> [w449]
    shift-right: [w445] -> _
    shift-left: 0 ("x") -> [w446]
    shift-right: [w441] -> _
    shift-left: T8 {"Array"=[], "Array"=[], "Array"=[], "Array"=[], "Array"=[], "Array"=[], "Array"=[], "Array"=[]} -> [w448]
    stop <- "stop" stop-if-true
    n195 = call-poly <instrlib>:"niScope Fetch (poly).vi"("timeout"=0.0, "error in"=w462, "numSamples"=w458, "channels"=w459, "instrument handle"=w463) -> ("error out"=w456:errorcluster, "wfm"=w450:i16[][], "wfm info"=w451:T12, "instrument handle out"=w461:refnum<k15>)  [unwired: 3 in]
    n196 = Greater?(x="Reset Value attempt 2", y=w446) -> (0:w442:bool)
    n197 = And(x="Plot Data attempt 2", y=w442) -> (x .and. y?=w443:bool)
    n198 = case shown="True" w443 {
      tunnel: w449 -> [_ w473]
      tunnel: w451 -> [_ w472]
      tunnel: w450 -> [_ w471]
      tunnel: [T8 {"Array"=[], "Array"=[], "Array"=[], "Array"=[], "Array"=[], "Array"=[], "Array"=[], "Array"=[]} w470] -> w441
      tunnel: w448 -> [_ w469]
      tunnel: [0 ("x") w468] -> w445
      tunnel: w446 -> [_ w467]
      frame False {
      }
      frame True {
        n199 = case shown="8" w473 {
          tunnel: w472 -> [w510 w544 w575 w603 w604 w629 w669 w685]
          tunnel: w471 -> [w509 w543 w574 w602 w628 w650 w668 w684]
          tunnel: [w500 w535 w567 w596 w623 w646 w665 w682] -> w466
          tunnel: [w499 w534 w566 w595 w622 w645 w664 w681] -> w470
          tunnel: w469 -> [w498 w533 w565 w594 w621 w644 w663 w680]
          frame 8 {
            n200 = Unbundle(w498) -> ("Array"=w497:dbl[], "Array"=w496:dbl[], "Array"=w495:dbl[], "Array"=w494:dbl[], "Array"=w493:dbl[], "Array"=w492:dbl[], "Array"=w491:dbl[], "Array"=w490:dbl[])
            n201 = call "StandAloneTransient_SingleGraphCreation_DataCollection_Light.vi"("wfm"=w509, "index"=0, "wfm info"=w510) -> ("Array"=w482:dbl[])  [unwired: 8 in]
            n202 = call "StandAloneTransient_SingleGraphCreation_DataCollection_Light.vi"("wfm"=w509, "index"=1, "wfm info"=w510) -> ("Array"=w483:dbl[])  [unwired: 8 in]
            n203 = call "StandAloneTransient_SingleGraphCreation_DataCollection_Light.vi"("wfm"=w509, "index"=2, "wfm info"=w510) -> ("Array"=w484:dbl[])  [unwired: 8 in]
            n204 = call "StandAloneTransient_SingleGraphCreation_DataCollection_Light.vi"("wfm"=w509, "index"=3, "wfm info"=w510) -> ("Array"=w485:dbl[])  [unwired: 8 in]
            n205 = call "StandAloneTransient_SingleGraphCreation_DataCollection_Light.vi"("wfm"=w509, "index"=4, "wfm info"=w510) -> ("Array"=w486:dbl[])  [unwired: 8 in]
            n206 = call "StandAloneTransient_SingleGraphCreation_DataCollection_Light.vi"("wfm"=w509, "index"=5, "wfm info"=w510) -> ("Array"=w487:dbl[])  [unwired: 8 in]
            n207 = call "StandAloneTransient_SingleGraphCreation_DataCollection_Light.vi"("wfm"=w509, "index"=6, "wfm info"=w510) -> ("Array"=w488:dbl[])  [unwired: 8 in]
            n208 = call "StandAloneTransient_SingleGraphCreation_DataCollection_Light.vi"("wfm"=w509, "index"=7, "wfm info"=w510) -> ("Array"=w489:dbl[])  [unwired: 8 in]
            n209 = Insert Into Array(array=w497, new element=w482) -> (w481:dbl[])  [unwired: 1 in]
            n210 = Insert Into Array(array=w496, new element=w483) -> (w480:dbl[])  [unwired: 1 in]
            n211 = Insert Into Array(array=w495, new element=w484) -> (w479:dbl[])  [unwired: 1 in]
            n212 = Insert Into Array(array=w494, new element=w485) -> (w478:dbl[])  [unwired: 1 in]
            n213 = Insert Into Array(array=w493, new element=w486) -> (w477:dbl[])  [unwired: 1 in]
            n214 = Insert Into Array(array=w492, new element=w487) -> (w476:dbl[])  [unwired: 1 in]
            n215 = Insert Into Array(array=w491, new element=w488) -> (w475:dbl[])  [unwired: 1 in]
            n216 = Insert Into Array(array=w490, new element=w489) -> (w474:dbl[])  [unwired: 1 in]
            n217 = local write "Channel Graph 0"(w481) -> ()
            n218 = local write "Channel Graph 1"(w480) -> ()
            n219 = local write "Channel Graph 3"(w478) -> ()
            n220 = local write "Channel Graph 2"(w479) -> ()
            n221 = local write "Channel Graph 4"(w477) -> ()
            n222 = local write "Channel Graph 5"(w476) -> ()
            n223 = local write "Channel Graph 7"(w474) -> ()
            n224 = local write "Channel Graph 6"(w475) -> ()
            n225 = Build Array(w482, w483, w484, w485, w486, w487, w488, w489) -> (w500:dbl[][])
            n226 = Bundle("Array"=w481, "Array"=w480, "Array"=w479, "Array"=w478, "Array"=w477, "Array"=w476, "Array"=w475, "Array"=w474) -> (w499:T8)  [unwired: 1 in]
          }
          frame 7 {
            n227 = Unbundle(w533) -> ("Array"=w532:dbl[], "Array"=w531:dbl[], "Array"=w530:dbl[], "Array"=w529:dbl[], "Array"=w528:dbl[], "Array"=w527:dbl[], "Array"=w526:dbl[], "Array"=w511:dbl[])
            n228 = call "StandAloneTransient_SingleGraphCreation_DataCollection_Light.vi"("wfm"=w543, "index"=0, "wfm info"=w544) -> ("Array"=w519:dbl[])  [unwired: 8 in]
            n229 = call "StandAloneTransient_SingleGraphCreation_DataCollection_Light.vi"("wfm"=w543, "index"=1, "wfm info"=w544) -> ("Array"=w520:dbl[])  [unwired: 8 in]
            n230 = call "StandAloneTransient_SingleGraphCreation_DataCollection_Light.vi"("wfm"=w543, "index"=2, "wfm info"=w544) -> ("Array"=w521:dbl[])  [unwired: 8 in]
            n231 = call "StandAloneTransient_SingleGraphCreation_DataCollection_Light.vi"("wfm"=w543, "index"=3, "wfm info"=w544) -> ("Array"=w522:dbl[])  [unwired: 8 in]
            n232 = call "StandAloneTransient_SingleGraphCreation_DataCollection_Light.vi"("wfm"=w543, "index"=4, "wfm info"=w544) -> ("Array"=w523:dbl[])  [unwired: 8 in]
            n233 = call "StandAloneTransient_SingleGraphCreation_DataCollection_Light.vi"("wfm"=w543, "index"=5, "wfm info"=w544) -> ("Array"=w524:dbl[])  [unwired: 8 in]
            n234 = call "StandAloneTransient_SingleGraphCreation_DataCollection_Light.vi"("wfm"=w543, "index"=6, "wfm info"=w544) -> ("Array"=w525:dbl[])  [unwired: 8 in]
            n235 = Insert Into Array(array=w532, new element=w519) -> (w518:dbl[])  [unwired: 1 in]
            n236 = Insert Into Array(array=w531, new element=w520) -> (w517:dbl[])  [unwired: 1 in]
            n237 = Insert Into Array(array=w530, new element=w521) -> (w516:dbl[])  [unwired: 1 in]
            n238 = Insert Into Array(array=w529, new element=w522) -> (w515:dbl[])  [unwired: 1 in]
            n239 = Insert Into Array(array=w528, new element=w523) -> (w514:dbl[])  [unwired: 1 in]
            n240 = Insert Into Array(array=w527, new element=w524) -> (w513:dbl[])  [unwired: 1 in]
            n241 = Insert Into Array(array=w526, new element=w525) -> (w512:dbl[])  [unwired: 1 in]
            n242 = Build Array(w519, w520, w521, w522, w523, w524, w525) -> (w535:dbl[][])
            n243 = local write "Channel Graph 0"(w518) -> ()
            n244 = local write "Channel Graph 1"(w517) -> ()
            n245 = local write "Channel Graph 2"(w516) -> ()
            n246 = local write "Channel Graph 4"(w514) -> ()
            n247 = local write "Channel Graph 3"(w515) -> ()
            n248 = local write "Channel Graph 5"(w513) -> ()
            n249 = local write "Channel Graph 6"(w512) -> ()
            n250 = Bundle("Array"=w518, "Array"=w517, "Array"=w516, "Array"=w515, "Array"=w514, "Array"=w513, "Array"=w512, "Array"=w511) -> (w534:T8)  [unwired: 1 in]
          }
          frame 6 {
            n251 = Unbundle(w565) -> ("Array"=w564:dbl[], "Array"=w563:dbl[], "Array"=w562:dbl[], "Array"=w561:dbl[], "Array"=w560:dbl[], "Array"=w559:dbl[], "Array"=w546:dbl[], "Array"=w545:dbl[])
            n252 = call "StandAloneTransient_SingleGraphCreation_DataCollection_Light.vi"("wfm"=w574, "index"=0, "wfm info"=w575) -> ("Array"=w553:dbl[])  [unwired: 8 in]
            n253 = call "StandAloneTransient_SingleGraphCreation_DataCollection_Light.vi"("wfm"=w574, "index"=1, "wfm info"=w575) -> ("Array"=w554:dbl[])  [unwired: 8 in]
            n254 = call "StandAloneTransient_SingleGraphCreation_DataCollection_Light.vi"("wfm"=w574, "index"=2, "wfm info"=w575) -> ("Array"=w555:dbl[])  [unwired: 8 in]
            n255 = call "StandAloneTransient_SingleGraphCreation_DataCollection_Light.vi"("wfm"=w574, "index"=3, "wfm info"=w575) -> ("Array"=w556:dbl[])  [unwired: 8 in]
            n256 = call "StandAloneTransient_SingleGraphCreation_DataCollection_Light.vi"("wfm"=w574, "index"=4, "wfm info"=w575) -> ("Array"=w557:dbl[])  [unwired: 8 in]
            n257 = call "StandAloneTransient_SingleGraphCreation_DataCollection_Light.vi"("wfm"=w574, "index"=5, "wfm info"=w575) -> ("Array"=w558:dbl[])  [unwired: 8 in]
            n258 = Insert Into Array(array=w564, new element=w553) -> (w552:dbl[])  [unwired: 1 in]
            n259 = Insert Into Array(array=w563, new element=w554) -> (w551:dbl[])  [unwired: 1 in]
            n260 = Insert Into Array(array=w562, new element=w555) -> (w550:dbl[])  [unwired: 1 in]
            n261 = Insert Into Array(array=w561, new element=w556) -> (w549:dbl[])  [unwired: 1 in]
            n262 = Insert Into Array(array=w560, new element=w557) -> (w548:dbl[])  [unwired: 1 in]
            n263 = Insert Into Array(array=w559, new element=w558) -> (w547:dbl[])  [unwired: 1 in]
            n264 = Build Array(w553, w554, w555, w556, w557, w558) -> (w567:dbl[][])
            n265 = local write "Channel Graph 0"(w552) -> ()
            n266 = local write "Channel Graph 1"(w551) -> ()
            n267 = local write "Channel Graph 2"(w550) -> ()
            n268 = local write "Channel Graph 4"(w548) -> ()
            n269 = local write "Channel Graph 3"(w549) -> ()
            n270 = local write "Channel Graph 5"(w547) -> ()
            n271 = Bundle("Array"=w552, "Array"=w551, "Array"=w550, "Array"=w549, "Array"=w548, "Array"=w547, "Array"=w546, "Array"=w545) -> (w566:T8)  [unwired: 1 in]
          }
          frame 5 {
            n272 = Unbundle(w594) -> ("Array"=w593:dbl[], "Array"=w592:dbl[], "Array"=w591:dbl[], "Array"=w590:dbl[], "Array"=w589:dbl[], "Array"=w578:dbl[], "Array"=w577:dbl[], "Array"=w576:dbl[])
            n273 = call "StandAloneTransient_SingleGraphCreation_DataCollection_Light.vi"("wfm"=w602, "index"=0, "wfm info"=w603) -> ("Array"=w584:dbl[])  [unwired: 8 in]
            n274 = call "StandAloneTransient_SingleGraphCreation_DataCollection_Light.vi"("wfm"=w602, "index"=1, "wfm info"=w603) -> ("Array"=w585:dbl[])  [unwired: 8 in]
            n275 = call "StandAloneTransient_SingleGraphCreation_DataCollection_Light.vi"("wfm"=w602, "index"=2, "wfm info"=w603) -> ("Array"=w586:dbl[])  [unwired: 8 in]
            n276 = call "StandAloneTransient_SingleGraphCreation_DataCollection_Light.vi"("wfm"=w602, "index"=3, "wfm info"=w603) -> ("Array"=w587:dbl[])  [unwired: 8 in]
            n277 = call "StandAloneTransient_SingleGraphCreation_DataCollection_Light.vi"("wfm"=w602, "index"=4, "wfm info"=w603) -> ("Array"=w588:dbl[])  [unwired: 8 in]
            n278 = Insert Into Array(array=w593, new element=w584) -> (w583:dbl[])  [unwired: 1 in]
            n279 = Insert Into Array(array=w592, new element=w585) -> (w582:dbl[])  [unwired: 1 in]
            n280 = Insert Into Array(array=w591, new element=w586) -> (w581:dbl[])  [unwired: 1 in]
            n281 = Insert Into Array(array=w590, new element=w587) -> (w580:dbl[])  [unwired: 1 in]
            n282 = Insert Into Array(array=w589, new element=w588) -> (w579:dbl[])  [unwired: 1 in]
            n283 = Build Array(w584, w585, w586, w587, w588) -> (w596:dbl[][])
            n284 = local write "Channel Graph 0"(w583) -> ()
            n285 = local write "Channel Graph 1"(w582) -> ()
            n286 = local write "Channel Graph 2"(w581) -> ()
            n287 = local write "Channel Graph 4"(w579) -> ()
            n288 = local write "Channel Graph 3"(w580) -> ()
            n289 = Bundle("Array"=w583, "Array"=w582, "Array"=w581, "Array"=w580, "Array"=w579, "Array"=w578, "Array"=w577, "Array"=w576) -> (w595:T8)  [unwired: 1 in]
          }
          frame 4 {
            n290 = Unbundle(w621) -> ("Array"=w620:dbl[], "Array"=w619:dbl[], "Array"=w618:dbl[], "Array"=w617:dbl[], "Array"=w608:dbl[], "Array"=w607:dbl[], "Array"=w606:dbl[], "Array"=w605:dbl[])
            n291 = call "StandAloneTransient_SingleGraphCreation_DataCollection_Light.vi"("wfm"=w628, "index"=0, "wfm info"=w604) -> ("Array"=w613:dbl[])  [unwired: 8 in]
            n292 = call "StandAloneTransient_SingleGraphCreation_DataCollection_Light.vi"("wfm"=w628, "index"=1, "wfm info"=w604) -> ("Array"=w614:dbl[])  [unwired: 8 in]
            n293 = call "StandAloneTransient_SingleGraphCreation_DataCollection_Light.vi"("wfm"=w628, "index"=2, "wfm info"=w604) -> ("Array"=w615:dbl[])  [unwired: 8 in]
            n294 = call "StandAloneTransient_SingleGraphCreation_DataCollection_Light.vi"("wfm"=w628, "index"=3, "wfm info"=w604) -> ("Array"=w616:dbl[])  [unwired: 8 in]
            n295 = Insert Into Array(array=w620, new element=w613) -> (w612:dbl[])  [unwired: 1 in]
            n296 = Insert Into Array(array=w619, new element=w614) -> (w611:dbl[])  [unwired: 1 in]
            n297 = Insert Into Array(array=w618, new element=w615) -> (w610:dbl[])  [unwired: 1 in]
            n298 = Insert Into Array(array=w617, new element=w616) -> (w609:dbl[])  [unwired: 1 in]
            n299 = Build Array(w613, w614, w615, w616) -> (w623:dbl[][])
            n300 = local write "Channel Graph 0"(w612) -> ()
            n301 = local write "Channel Graph 1"(w611) -> ()
            n302 = local write "Channel Graph 2"(w610) -> ()
            n303 = local write "Channel Graph 3"(w609) -> ()
            n304 = Bundle("Array"=w612, "Array"=w611, "Array"=w610, "Array"=w609, "Array"=w608, "Array"=w607, "Array"=w606, "Array"=w605) -> (w622:T8)  [unwired: 1 in]
          }
          frame 3 {
            n305 = Unbundle(w644) -> ("Array"=w643:dbl[], "Array"=w642:dbl[], "Array"=w641:dbl[], "Array"=w634:dbl[], "Array"=w633:dbl[], "Array"=w632:dbl[], "Array"=w631:dbl[], "Array"=w630:dbl[])
            n306 = call "StandAloneTransient_SingleGraphCreation_DataCollection_Light.vi"("wfm"=w650, "index"=0, "wfm info"=w629) -> ("Array"=w638:dbl[])  [unwired: 8 in]
            n307 = call "StandAloneTransient_SingleGraphCreation_DataCollection_Light.vi"("wfm"=w650, "index"=1, "wfm info"=w629) -> ("Array"=w639:dbl[])  [unwired: 8 in]
            n308 = call "StandAloneTransient_SingleGraphCreation_DataCollection_Light.vi"("wfm"=w650, "index"=2, "wfm info"=w629) -> ("Array"=w640:dbl[])  [unwired: 8 in]
            n309 = Insert Into Array(array=w643, new element=w638) -> (w637:dbl[])  [unwired: 1 in]
            n310 = Insert Into Array(array=w642, new element=w639) -> (w636:dbl[])  [unwired: 1 in]
            n311 = Insert Into Array(array=w641, new element=w640) -> (w635:dbl[])  [unwired: 1 in]
            n312 = local write "Channel Graph 0"(w637) -> ()
            n313 = local write "Channel Graph 1"(w636) -> ()
            n314 = local write "Channel Graph 2"(w635) -> ()
            n315 = Build Array(w638, w639, w640) -> (w646:dbl[][])
            n316 = Bundle("Array"=w637, "Array"=w636, "Array"=w635, "Array"=w634, "Array"=w633, "Array"=w632, "Array"=w631, "Array"=w630) -> (w645:T8)  [unwired: 1 in]
          }
          frame 2 {
            n317 = Unbundle(w663) -> ("Array"=w662:dbl[], "Array"=w661:dbl[], "Array"=w656:dbl[], "Array"=w655:dbl[], "Array"=w654:dbl[], "Array"=w653:dbl[], "Array"=w652:dbl[], "Array"=w651:dbl[])
            n318 = call "StandAloneTransient_SingleGraphCreation_DataCollection_Light.vi"("wfm"=w668, "index"=0, "wfm info"=w669) -> ("Array"=w659:dbl[])  [unwired: 8 in]
            n319 = call "StandAloneTransient_SingleGraphCreation_DataCollection_Light.vi"("wfm"=w668, "index"=1, "wfm info"=w669) -> ("Array"=w660:dbl[])  [unwired: 8 in]
            n320 = Insert Into Array(array=w662, new element=w659) -> (w658:dbl[])  [unwired: 1 in]
            n321 = Insert Into Array(array=w661, new element=w660) -> (w657:dbl[])  [unwired: 1 in]
            n322 = Build Array(w659, w660) -> (w665:dbl[][])
            n323 = local write "Channel Graph 0"(w658) -> ()
            n324 = local write "Channel Graph 1"(w657) -> ()
            n325 = Bundle("Array"=w658, "Array"=w657, "Array"=w656, "Array"=w655, "Array"=w654, "Array"=w653, "Array"=w652, "Array"=w651) -> (w664:T8)  [unwired: 1 in]
          }
          frame 1, Default {
            n326 = Unbundle(w680) -> ("Array"=w679:dbl[], "Array"=w676:dbl[], "Array"=w675:dbl[], "Array"=w674:dbl[], "Array"=w673:dbl[], "Array"=w672:dbl[], "Array"=w671:dbl[], "Array"=w670:dbl[])
            n327 = call "StandAloneTransient_SingleGraphCreation_DataCollection_Light.vi"("wfm"=w684, "index"=0, "wfm info"=w685) -> ("Array"=w678:dbl[])  [unwired: 8 in]
            n328 = Insert Into Array(array=w679, new element=w678) -> (w677:dbl[])  [unwired: 1 in]
            n329 = Build Array(w678) -> (w682:dbl[][])
            n330 = local write "Channel Graph 0"(w677) -> ()
            n331 = Bundle("Array"=w677, "Array"=w676, "Array"=w675, "Array"=w674, "Array"=w673, "Array"=w672, "Array"=w671, "Array"=w670) -> (w681:T8)  [unwired: 1 in]
          }
        }
        "Pryor's Graph" <- w466
        n332 = Increment(x=w467) -> (x+1=w468:i32)
      }
    }
    n333 = Bundle(cluster=T9 {"wfm info"=[], "wfm"=[]}, "wfm info"=w451, "wfm"=w450) -> (w454:T9)
    n334 = Enqueue Element(queue=w455, element=w454, error in (no error)=w456) -> (error out=w452:errorcluster)  [unwired: 1 in, 2 out]
    "end record" <- "stop"
  }
  n335 = Array Size(array=w8) -> (size(s)=w15:i32)
  n336 = Greater?(x=w15, y=1) -> (0:w14:bool)
  n337 = case shown="False" w14 {
    tunnel: w8 -> [w689 w693]
    tunnel: w15 -> [w687 w691]
    tunnel: [w686 w690] -> w17
    frame False {
      n338 = Array Subset(array=w689, index=0, length=w687) -> (w686:refnum<file>[])
    }
    frame True {
      n339 = Array Subset(array=w693, index=1, length=w691) -> (w690:refnum<file>[])
    }
  }
  n340 = Close File(refnum=w6, error in=w11) -> (error out=w12:errorcluster)  [unwired: 1 out]
  n341 = for {
    tunnel: w9 -> [w696] mode=indexing
    shift-right: [w695] -> w16
    shift-left: w12 -> [w694]
    n342 = Close File(refnum=w696, error in=w694) -> (error out=w695:errorcluster)  [unwired: 1 out]
  }
  n343 = for {
    tunnel: w17 -> [w698] mode=indexing
    shift-right: [w697] -> w10
    shift-left: w16 -> [w699]
    n344 = Close File(refnum=w698, error in=w699) -> (error out=w697:errorcluster)  [unwired: 1 out]
  }
  n345 = Merge Errors(w79, w10) -> (w78:errorcluster)
  n346 = call <instrlib>:"niScope Close.vi"("instrument handle"=w84, "error in"=w78) -> ("error out"=→"error out":errorcluster)  [unwired: 13 in]
